vi "Main.vi"(11 "Module Admin":refnum<class "Delacor_lib_QMH_Module Admin.lvclass">) -> ()   [LabVIEW 2021, in "Host Main.lvlib"]
doc: "This template is based off of the Queued Message Handler design pattern and the Queued Message Handler project template that ships with LabVIEW.\n\nThe main difference is that the queue is private to this module and communication between modules is performed via Broadcast and Request events.\n\nRequest events are wrapped in public API methods and are handled in the Event Handling Loop (EHL) of this VI. Any module can register for Broadcast events sent by this module. The EHL generates messages based on user interface actions.\n\nThe Message Handling Loop (MHL) processes messages generated by the EHL, or by other messages. The messages are string values, so new messages can be added easily to the Message Cases case structure in the MHL. Each message cluster can also provide an optional value for Message Data, which is a variant that can be converted to whatever message-specific data is required.\n_____\nBased on DQMH Project Template 7.0.1.1316."
uses:
  Host Main.lvlib
  <vilib>/Delacor/Delacor QMH/Libraries/Module Admin_class/Delacor_lib_QMH_Module Admin.lvclass
  Analog Output/Controls/AO JSON Data Cluster.ctl
  Analog Output/Controls/AO Interface Data Cluster.ctl
  Analog Output/Controls/AO Channel Configuration Cluster.ctl
  Analog Output/Controls/AO Timing Cluster.ctl
  Digital Output/Controls/DIO Configuration cluster.ctl
  Digital Output/Controls/DIO Interface Data.ctl
  Digital Output/SubVIs/Digital Dynamic Cluster.ctl
  Module Data--cluster.ctl
  Host/Controls/Host - GUI Data Cluster.ctl
  Host/Async JSON Cluster.ctl
  Host/Async Interface Data Cluster.ctl
  Async Serial/Controls/Async Serial Configuration Cluster.ctl
  Async Serial/Controls/Async Frame Info Cluster.ctl
  Async Serial/Controls/Async Message Info Cluster.ctl
  Host/Controls/Host Data Cluster.ctl
  Main Engine/Controls/Main Engine CPU Info.ctl
  <vilib>/Wovalab/Utilities/Helper Loop Periodic Timing/Helper Loop Periodic Timing.lvclass/Helper Loop Periodic Timing.ctl
  Host-Control's/Module ID Action Enum.ctl
  Host-Control's/RT Exec FGV Action.ctl
  <vilib>/Delacor/Delacor QMH/Libraries/Message Queue_class/Delacor_lib_QMH_Message Queue.lvclass/Delacor_lib_QMH_Message Queue.ctl
  Stop Argument--cluster.ctl
  <vilib>/Delacor/Delacor QMH/Libraries/Module Admin_class/Delacor_lib_QMH_Module Admin.lvclass/Delacor_lib_QMH_Module Admin.ctl
  <vilib>/Utility/miscctls.llb/LVPointTypeDef.ctl
  Launch RT Acq Argument--cluster.ctl
  Host-Control's/DTT Test folder Name's.ctl
  Host-Control's/HW Name Enum.ctl
  <vilib>/Delacor/Delacor QMH/Libraries/Message Queue_class/Delacor_lib_QMH_Enqueue Message (Single).vi
  <vilib>/Delacor/Delacor QMH/Libraries/Module Admin_class/Delacor_lib_QMH_Get External Launch.vi
  <vilib>/Wovalab/Utilities/Helper Loop Periodic Timing/U32 Max Value--constant.vi
  <vilib>/Wovalab/Utilities/Helper Loop Periodic Timing/Update Last Execution Time.vi
  <vilib>/addons/_JKI.lib/Serialization/JSON/Library/Flatten To JSON String.vi
  <vilib>/Wovalab/Utilities/Helper Loop Periodic Timing/Helper Loop Periodic Timing.lvclass
  <vilib>/Delacor/Delacor QMH/Libraries/Message Queue_class/Delacor_lib_QMH_Message Queue.lvclass
  RT Acquisition Engine/RT Acquisition Engine.lvlib
  Test Configuration/Test Configuration.lvlib
  Test Panel/Test Panel.lvlib
  Configuration/Configuration.lvlib
  Hardware Selection/Hardware Selection.lvlib
  <userlib>/_OpenG.lib/appcontrol/appcontrol.llb/openg_application_control.lvlib
  RT Acquisition Engine/Clone Registration/Clone Registration.lvlib
  TCP-IP Engine/Clone Registration/Clone Registration.lvlib
  TCP-IP Engine/TCP-IP Engine.lvlib
  AS-Configuration/AS-Configuration.lvlib
  <vilib>/Utility/TDMS File Viewer/NI_TDMS File Viewer.lvlib
  Safety/Safety.lvlib
panel:
  in  "Hardware Selection":bool
  in  "AI 2":T1[](array[typedef]) {"Interface Data"."Timing"."sample mode" items=["Finite Samples"=10178, "Continuous Samples"=10123, "Hardware Timed Single Point"=12522]}
  out "Capsule-4":bool
  out "Capsule-2":bool
  out "Capsule-1":bool
  in  "DO":T5[](array[typedef])=[{"Interface"="DIO", "Interface Data"={"Command"="Configure", "SubCmd"="DO", "Frequency"=500, "Data"=[{"Channel"="Mod1/port0/line0", "Data"=[0], "Identification Name"=""}, {"Channel"="Mod1/port0/line1", "Data"=[0], "Identification Name"=""}, {"Channel"="Mod1/port0/line2", "Data"=[0], "Identification Name"=""}, {"Channel"="Mod1/port0/line3", "Data"=[0], "Identification Name"=""}, {"Channel"="Mod1/port0/line4", "Data"=[0], "Identification Name"=""}, {"Channel"="Mod1/port0/line5", "Data"=[0], "Identification Name"=""}, {"Channel"="Mod1/port0/line6", "Data"=[0], "Identification Name"=""}, {"Channel"="Mod1/port0/line7", "Data"=[0], "Identification Name"=""}, {"Channel"="Mod1/port0/line8", "Data"=[0], "Identification Name"=""}, {"Channel"="Mod1/port0/line9", "Data"=[0], "Identification Name"=""}, {"Channel"="Mod1/port0/line10", "Data"=[0], "Identification Name"=""}, {"Channel"="Mod1/port0/line11", "Data"=[0], "Identification Name"=""}, {"Channel"="Mod1/port0/line12", "Data"=[0], "Identification Name"=""}, {"Channel"="Mod1/port0/line13", "Data"=[0], "Identification Name"=""}, {"Channel"="Mod1/port0/line14", "Data"=[0], "Identification Name"=""}, {"Channel"="Mod1/port0/line15", "Data"=[0], "Identification Name"=""}, {"Channel"="Mod1/port0/line16", "Data"=[0], "Identification Name"=""}, {"Channel"="Mod1/port0/line17", "Data"=[0], "Identification Name"=""}, {"Channel"="Mod1/port0/line18", "Data"=[0], "Identification Name"=""}, {"Channel"="Mod1/port0/line19", "Data"=[0], "Identification Name"=""}, {"Channel"="Mod1/port0/line20", "Data"=[0], "Identification Name"=""}, {"Channel"="Mod1/port0/line21", "Data"=[0], "Identification Name"=""}, {"Channel"="Mod1/port0/line22", "Data"=[0], "Identification Name"=""}, {"Channel"="Mod1/port0/line23", "Data"=[0], "Identification Name"=""}, {"Channel"="Mod1/port0/line24", "Data"=[0], "Identification Name"=""}, {"Channel"="Mod1/port0/line25", "Data"=[0], "Identification Name"=""}, {"Channel"="Mod1/port0/line26", "Data"=[0], "Identification Name"=""}, {"Channel"="Mod1/port0/line27", "Data"=[0], "Identification Name"=""}, {"Channel"="Mod1/port0/line28", "Data"=[0], "Identification Name"=""}, {"Channel"="Mod1/port0/line29", "Data"=[0], "Identification Name"=""}, {"Channel"="Mod1/port0/line30", "Data"=[0], "Identification Name"=""}, {"Channel"="Mod1/port0/line31", "Data"=[0], "Identification Name"=""}]}}, {"Interface"="DIO", "Interface Data"={"Command"="Configure", "SubCmd"="DO", "Frequency"=500, "Data"=[{"Channel"="Mod1/port0/line0", "Data"=[0], "Identification Name"=""}, {"Channel"="Mod1/port0/line1", "Data"=[0], "Identification Name"=""}, {"Channel"="Mod1/port0/line2", "Data"=[0], "Identification Name"=""}, {"Channel"="Mod1/port0/line3", "Data"=[0], "Identification Name"=""}, {"Channel"="Mod1/port0/line4", "Data"=[0], "Identification Name"=""}, {"Channel"="Mod1/port0/line5", "Data"=[0], "Identification Name"=""}, {"Channel"="Mod1/port0/line6", "Data"=[0], "Identification Name"=""}, {"Channel"="Mod1/port0/line7", "Data"=[0], "Identification Name"=""}, {"Channel"="Mod1/port0/line8", "Data"=[0], "Identification Name"=""}, {"Channel"="Mod1/port0/line9", "Data"=[0], "Identification Name"=""}, {"Channel"="Mod1/port0/line10", "Data"=[0], "Identification Name"=""}, {"Channel"="Mod1/port0/line11", "Data"=[0], "Identification Name"=""}, {"Channel"="Mod1/port0/line12", "Data"=[0], "Identification Name"=""}, {"Channel"="Mod1/port0/line13", "Data"=[0], "Identification Name"=""}, {"Channel"="Mod1/port0/line14", "Data"=[0], "Identification Name"=""}, {"Channel"="Mod1/port0/line15", "Data"=[0], "Identification Name"=""}, {"Channel"="Mod1/port0/line16", "Data"=[0], "Identification Name"=""}, {"Channel"="Mod1/port0/line17", "Data"=[0], "Identification Name"=""}, {"Channel"="Mod1/port0/line18", "Data"=[0], "Identification Name"=""}, {"Channel"="Mod1/port0/line19", "Data"=[0], "Identification Name"=""}, {"Channel"="Mod1/port0/line20", "Data"=[0], "Identification Name"=""}, {"Channel"="Mod1/port0/line21", "Data"=[0], "Identification Name"=""}, {"Channel"="Mod1/port0/line22", "Data"=[0], "Identification Name"=""}, {"Channel"="Mod1/port0/line23", "Data"=[0], "Identification Name"=""}, {"Channel"="Mod1/port0/line24", "Data"=[0], "Identification Name"=""}, {"Channel"="Mod1/port0/line25", "Data"=[0], "Identification Name"=""}, {"Channel"="Mod1/port0/line26", "Data"=[0], "Identification Name"=""}, {"Channel"="Mod1/port0/line27", "Data"=[0], "Identification Name"=""}, {"Channel"="Mod1/port0/line28", "Data"=[0], "Identification Name"=""}, {"Channel"="Mod1/port0/line29", "Data"=[0], "Identification Name"=""}, {"Channel"="Mod1/port0/line30", "Data"=[0], "Identification Name"=""}, {"Channel"="Mod1/port0/line31", "Data"=[0], "Identification Name"=""}, {"Channel"="Mod2/port0/line0", "Data"=[0], "Identification Name"=""}, {"Channel"="Mod2/port0/line1", "Data"=[0], "Identification Name"=""}, {"Channel"="Mod2/port0/line2", "Data"=[0], "Identification Name"=""}, {"Channel"="Mod2/port0/line3", "Data"=[0], "Identification Name"=""}, {"Channel"="Mod2/port0/line4", "Data"=[0], "Identification Name"=""}, {"Channel"="Mod2/port0/line5", "Data"=[0], "Identification Name"=""}, {"Channel"="Mod2/port0/line6", "Data"=[0], "Identification Name"=""}, {"Channel"="Mod2/port0/line7", "Data"=[0], "Identification Name"=""}, {"Channel"="Mod2/port0/line8", "Data"=[0], "Identification Name"=""}]}}, {"Interface"="DIO", "Interface Data"={"Command"="Configure", "SubCmd"="DO", "Frequency"=500, "Data"=[{"Channel"="Mod1/port0/line0", "Data"=[0], "Identification Name"=""}, {"Channel"="Mod1/port0/line1", "Data"=[0], "Identification Name"=""}, {"Channel"="Mod1/port0/line2", "Data"=[0], "Identification Name"=""}, {"Channel"="Mod1/port0/line3", "Data"=[0], "Identification Name"=""}, {"Channel"="Mod1/port0/line4", "Data"=[0], "Identification Name"=""}, {"Channel"="Mod1/port0/line5", "Data"=[0], "Identification Name"=""}, {"Channel"="Mod1/port0/line6", "Data"=[], "Identification Name"=""}, {"Channel"="Mod1/port0/line7", "Data"=[0], "Identification Name"=""}, {"Channel"="Mod1/port0/line8", "Data"=[0], "Identification Name"=""}, {"Channel"="Mod1/port0/line9", "Data"=[0], "Identification Name"=""}, {"Channel"="Mod1/port0/line10", "Data"=[0], "Identification Name"=""}, {"Channel"="Mod1/port0/line11", "Data"=[0], "Identification Name"=""}, {"Channel"="Mod1/port0/line12", "Data"=[0], "Identification Name"=""}, {"Channel"="Mod1/port0/line13", "Data"=[0], "Identification Name"=""}, {"Channel"="Mod1/port0/line14", "Data"=[0], "Identification Name"=""}, {"Channel"="Mod1/port0/line15", "Data"=[0], "Identification Name"=""}, {"Channel"="Mod1/port0/line16", "Data"=[0], "Identification Name"=""}, {"Channel"="Mod1/port0/line17", "Data"=[0], "Identification Name"=""}, {"Channel"="Mod1/port0/line18", "Data"=[0], "Identification Name"=""}, {"Channel"="Mod1/port0/line19", "Data"=[0], "Identification Name"=""}, {"Channel"="Mod1/port0/line20", "Data"=[0], "Identification Name"=""}, {"Channel"="Mod1/port0/line21", "Data"=[0], "Identification Name"=""}, {"Channel"="Mod1/port0/line22", "Data"=[0], "Identification Name"=""}, {"Channel"="Mod1/port0/line23", "Data"=[0], "Identification Name"=""}, {"Channel"="Mod1/port0/line24", "Data"=[0], "Identification Name"=""}, {"Channel"="Mod1/port0/line25", "Data"=[0], "Identification Name"=""}, {"Channel"="Mod1/port0/line26", "Data"=[0], "Identification Name"=""}, {"Channel"="Mod1/port0/line27", "Data"=[0], "Identification Name"=""}, {"Channel"="Mod1/port0/line28", "Data"=[0], "Identification Name"=""}, {"Channel"="Mod1/port0/line29", "Data"=[0], "Identification Name"=""}, {"Channel"="Mod1/port0/line30", "Data"=[0], "Identification Name"=""}, {"Channel"="Mod1/port0/line31", "Data"=[0], "Identification Name"=""}]}}, {"Interface"="DIO", "Interface Data"={"Command"="Configure", "SubCmd"="DO", "Frequency"=500, "Data"=[{"Channel"="Mod1/port0/line0", "Data"=[0], "Identification Name"=""}, {"Channel"="Mod1/port0/line1", "Data"=[0], "Identification Name"=""}, {"Channel"="Mod1/port0/line2", "Data"=[0], "Identification Name"=""}, {"Channel"="Mod1/port0/line3", "Data"=[0], "Identification Name"=""}, {"Channel"="Mod1/port0/line4", "Data"=[0], "Identification Name"=""}, {"Channel"="Mod1/port0/line5", "Data"=[0], "Identification Name"=""}, {"Channel"="Mod1/port0/line6", "Data"=[0], "Identification Name"=""}, {"Channel"="Mod1/port0/line7", "Data"=[0], "Identification Name"=""}, {"Channel"="Mod1/port0/line8", "Data"=[0], "Identification Name"=""}, {"Channel"="Mod1/port0/line9", "Data"=[0], "Identification Name"=""}, {"Channel"="Mod1/port0/line10", "Data"=[0], "Identification Name"=""}, {"Channel"="Mod1/port0/line11", "Data"=[0], "Identification Name"=""}, {"Channel"="Mod1/port0/line12", "Data"=[0], "Identification Name"=""}, {"Channel"="Mod1/port0/line13", "Data"=[0], "Identification Name"=""}, {"Channel"="Mod1/port0/line14", "Data"=[0], "Identification Name"=""}, {"Channel"="Mod1/port0/line15", "Data"=[0], "Identification Name"=""}, {"Channel"="Mod1/port0/line16", "Data"=[0], "Identification Name"=""}, {"Channel"="Mod1/port0/line17", "Data"=[0], "Identification Name"=""}, {"Channel"="Mod1/port0/line18", "Data"=[0], "Identification Name"=""}, {"Channel"="Mod1/port0/line19", "Data"=[0], "Identification Name"=""}, {"Channel"="Mod1/port0/line20", "Data"=[0], "Identification Name"=""}, {"Channel"="Mod1/port0/line21", "Data"=[0], "Identification Name"=""}, {"Channel"="Mod1/port0/line22", "Data"=[0], "Identification Name"=""}, {"Channel"="Mod1/port0/line23", "Data"=[0], "Identification Name"=""}, {"Channel"="Mod1/port0/line24", "Data"=[0], "Identification Name"=""}, {"Channel"="Mod1/port0/line25", "Data"=[0], "Identification Name"=""}, {"Channel"="Mod1/port0/line26", "Data"=[0], "Identification Name"=""}, {"Channel"="Mod1/port0/line27", "Data"=[0], "Identification Name"=""}, {"Channel"="Mod1/port0/line28", "Data"=[0], "Identification Name"=""}, {"Channel"="Mod1/port0/line29", "Data"=[0], "Identification Name"=""}, {"Channel"="Mod1/port0/line30", "Data"=[0], "Identification Name"=""}, {"Channel"="Mod1/port0/line31", "Data"=[0], "Identification Name"=""}]}}, {"Interface"="DIO", "Interface Data"={"Command"="Configure", "SubCmd"="DO", "Frequency"=500, "Data"=[{"Channel"="Mod1/port0/line0", "Data"=[0], "Identification Name"=""}, {"Channel"="Mod1/port0/line1", "Data"=[0], "Identification Name"=""}, {"Channel"="Mod1/port0/line2", "Data"=[0], "Identification Name"=""}, {"Channel"="Mod1/port0/line3", "Data"=[0], "Identification Name"=""}, {"Channel"="Mod1/port0/line4", "Data"=[0], "Identification Name"=""}, {"Channel"="Mod1/port0/line5", "Data"=[0], "Identification Name"=""}, {"Channel"="Mod1/port0/line6", "Data"=[0], "Identification Name"=""}, {"Channel"="Mod1/port0/line7", "Data"=[0], "Identification Name"=""}, {"Channel"="Mod1/port0/line8", "Data"=[0], "Identification Name"=""}, {"Channel"="Mod1/port0/line9", "Data"=[0], "Identification Name"=""}, {"Channel"="Mod1/port0/line10", "Data"=[0], "Identification Name"=""}, {"Channel"="Mod1/port0/line11", "Data"=[0], "Identification Name"=""}, {"Channel"="Mod1/port0/line12", "Data"=[0], "Identification Name"=""}, {"Channel"="Mod1/port0/line13", "Data"=[0], "Identification Name"=""}, {"Channel"="Mod1/port0/line14", "Data"=[0], "Identification Name"=""}, {"Channel"="Mod1/port0/line15", "Data"=[0], "Identification Name"=""}, {"Channel"="Mod1/port0/line16", "Data"=[0], "Identification Name"=""}, {"Channel"="Mod1/port0/line17", "Data"=[0], "Identification Name"=""}, {"Channel"="Mod1/port0/line18", "Data"=[0], "Identification Name"=""}, {"Channel"="Mod1/port0/line19", "Data"=[0], "Identification Name"=""}, {"Channel"="Mod1/port0/line20", "Data"=[0], "Identification Name"=""}, {"Channel"="Mod1/port0/line21", "Data"=[0], "Identification Name"=""}, {"Channel"="Mod1/port0/line22", "Data"=[0], "Identification Name"=""}, {"Channel"="Mod1/port0/line23", "Data"=[0], "Identification Name"=""}, {"Channel"="Mod1/port0/line24", "Data"=[0], "Identification Name"=""}, {"Channel"="Mod1/port0/line25", "Data"=[0], "Identification Name"=""}, {"Channel"="Mod1/port0/line26", "Data"=[0], "Identification Name"=""}, {"Channel"="Mod1/port0/line27", "Data"=[0], "Identification Name"=""}, {"Channel"="Mod1/port0/line28", "Data"=[0], "Identification Name"=""}, {"Channel"="Mod1/port0/line29", "Data"=[0], "Identification Name"=""}, {"Channel"="Mod1/port0/line30", "Data"=[0], "Identification Name"=""}, {"Channel"="Mod1/port0/line31", "Data"=[0], "Identification Name"=""}]}}, {"Interface"="DIO", "Interface Data"={"Command"="Configure", "SubCmd"="DO", "Frequency"=500, "Data"=[{"Channel"="Mod1/port0/line0", "Data"=[0], "Identification Name"=""}, {"Channel"="Mod1/port0/line1", "Data"=[0], "Identification Name"=""}, {"Channel"="Mod1/port0/line2", "Data"=[0], "Identification Name"=""}, {"Channel"="Mod1/port0/line3", "Data"=[0], "Identification Name"=""}, {"Channel"="Mod1/port0/line4", "Data"=[0], "Identification Name"=""}, {"Channel"="Mod1/port0/line5", "Data"=[0], "Identification Name"=""}, {"Channel"="Mod1/port0/line6", "Data"=[0], "Identification Name"=""}, {"Channel"="Mod1/port0/line7", "Data"=[0], "Identification Name"=""}, {"Channel"="Mod1/port0/line8", "Data"=[0], "Identification Name"=""}, {"Channel"="Mod1/port0/line9", "Data"=[0], "Identification Name"=""}, {"Channel"="Mod1/port0/line10", "Data"=[0], "Identification Name"=""}, {"Channel"="Mod1/port0/line11", "Data"=[0], "Identification Name"=""}, {"Channel"="Mod1/port0/line12", "Data"=[0], "Identification Name"=""}, {"Channel"="Mod1/port0/line13", "Data"=[0], "Identification Name"=""}, {"Channel"="Mod1/port0/line14", "Data"=[0], "Identification Name"=""}, {"Channel"="Mod1/port0/line15", "Data"=[0], "Identification Name"=""}, {"Channel"="Mod1/port0/line16", "Data"=[0], "Identification Name"=""}, {"Channel"="Mod1/port0/line17", "Data"=[0], "Identification Name"=""}, {"Channel"="Mod1/port0/line18", "Data"=[0], "Identification Name"=""}, {"Channel"="Mod1/port0/line19", "Data"=[0], "Identification Name"=""}, {"Channel"="Mod1/port0/line20", "Data"=[0], "Identification Name"=""}, {"Channel"="Mod1/port0/line21", "Data"=[0], "Identification Name"=""}, {"Channel"="Mod1/port0/line22", "Data"=[0], "Identification Name"=""}, {"Channel"="Mod1/port0/line23", "Data"=[0], "Identification Name"=""}, {"Channel"="Mod1/port0/line24", "Data"=[0], "Identification Name"=""}, {"Channel"="Mod1/port0/line25", "Data"=[0], "Identification Name"=""}, {"Channel"="Mod1/port0/line26", "Data"=[0], "Identification Name"=""}, {"Channel"="Mod1/port0/line27", "Data"=[0], "Identification Name"=""}, {"Channel"="Mod1/port0/line28", "Data"=[0], "Identification Name"=""}, {"Channel"="Mod1/port0/line29", "Data"=[0], "Identification Name"=""}, {"Channel"="Mod1/port0/line30", "Data"=[0], "Identification Name"=""}, {"Channel"="Mod1/port0/line31", "Data"=[0], "Identification Name"=""}, {"Channel"="Mod2/port0/line0", "Data"=[0], "Identification Name"=""}, {"Channel"="Mod2/port0/line1", "Data"=[0], "Identification Name"=""}, {"Channel"="Mod2/port0/line2", "Data"=[0], "Identification Name"=""}, {"Channel"="Mod2/port0/line3", "Data"=[0], "Identification Name"=""}, {"Channel"="Mod2/port0/line4", "Data"=[0], "Identification Name"=""}, {"Channel"="Mod2/port0/line5", "Data"=[0], "Identification Name"=""}, {"Channel"="Mod2/port0/line6", "Data"=[0], "Identification Name"=""}, {"Channel"="Mod2/port0/line7", "Data"=[0], "Identification Name"=""}, {"Channel"="Mod2/port0/line8", "Data"=[0], "Identification Name"=""}, {"Channel"="Mod2/port0/line9", "Data"=[0], "Identification Name"=""}, {"Channel"="Mod2/port0/line10", "Data"=[0], "Identification Name"=""}, {"Channel"="Mod2/port0/line11", "Data"=[0], "Identification Name"=""}, {"Channel"="Mod2/port0/line12", "Data"=[0], "Identification Name"=""}, {"Channel"="Mod2/port0/line13", "Data"=[0], "Identification Name"=""}, {"Channel"="Mod2/port0/line14", "Data"=[0], "Identification Name"=""}, {"Channel"="Mod2/port0/line15", "Data"=[0], "Identification Name"=""}, {"Channel"="Mod2/port0/line16", "Data"=[0], "Identification Name"=""}, {"Channel"="Mod2/port0/line17", "Data"=[0], "Identification Name"=""}, {"Channel"="Mod2/port0/line18", "Data"=[0], "Identification Name"=""}, {"Channel"="Mod2/port0/line19", "Data"=[0], "Identification Name"=""}, {"Channel"="Mod2/port0/line20", "Data"=[0], "Identification Name"=""}, {"Channel"="Mod2/port0/line21", "Data"=[0], "Identification Name"=""}, {"Channel"="Mod2/port0/line22", "Data"=[0], "Identification Name"=""}, {"Channel"="Mod2/port0/line23", "Data"=[0], "Identification Name"=""}, {"Channel"="Mod2/port0/line24", "Data"=[0], "Identification Name"=""}, {"Channel"="Mod2/port0/line25", "Data"=[0], "Identification Name"=""}, {"Channel"="Mod2/port0/line26", "Data"=[0], "Identification Name"=""}, {"Channel"="Mod2/port0/line27", "Data"=[0], "Identification Name"=""}, {"Channel"="Mod2/port0/line28", "Data"=[0], "Identification Name"=""}, {"Channel"="Mod2/port0/line29", "Data"=[0], "Identification Name"=""}, {"Channel"="Mod2/port0/line30", "Data"=[0], "Identification Name"=""}, {"Channel"="Mod2/port0/line31", "Data"=[0], "Identification Name"=""}]}}]
  in  "DI":T5[](array[typedef])=[{"Interface"="DIO", "Interface Data"={"Command"="Configure", "SubCmd"="DI", "Frequency"=500, "Data"=[{"Channel"="Mod3/port0/line0", "Data"=[0], "Identification Name"=""}, {"Channel"="Mod3/port0/line1", "Data"=[0], "Identification Name"=""}, {"Channel"="Mod3/port0/line2", "Data"=[0], "Identification Name"=""}, {"Channel"="Mod3/port0/line3", "Data"=[0], "Identification Name"=""}, {"Channel"="Mod3/port0/line4", "Data"=[0], "Identification Name"=""}, {"Channel"="Mod3/port0/line5", "Data"=[0], "Identification Name"=""}, {"Channel"="Mod3/port0/line6", "Data"=[0], "Identification Name"=""}, {"Channel"="Mod3/port0/line7", "Data"=[0], "Identification Name"=""}, {"Channel"="Mod3/port0/line8", "Data"=[0], "Identification Name"=""}, {"Channel"="Mod3/port0/line9", "Data"=[0], "Identification Name"=""}, {"Channel"="Mod3/port0/line10", "Data"=[0], "Identification Name"=""}, {"Channel"="Mod3/port0/line11", "Data"=[0], "Identification Name"=""}, {"Channel"="Mod3/port0/line12", "Data"=[0], "Identification Name"=""}, {"Channel"="Mod3/port0/line13", "Data"=[0], "Identification Name"=""}, {"Channel"="Mod3/port0/line14", "Data"=[0], "Identification Name"=""}, {"Channel"="Mod3/port0/line15", "Data"=[0], "Identification Name"=""}, {"Channel"="Mod3/port0/line16", "Data"=[0], "Identification Name"=""}, {"Channel"="Mod3/port0/line17", "Data"=[0], "Identification Name"=""}, {"Channel"="Mod3/port0/line18", "Data"=[0], "Identification Name"=""}, {"Channel"="Mod3/port0/line19", "Data"=[0], "Identification Name"=""}, {"Channel"="Mod3/port0/line20", "Data"=[0], "Identification Name"=""}, {"Channel"="Mod3/port0/line21", "Data"=[0], "Identification Name"=""}, {"Channel"="Mod3/port0/line22", "Data"=[0], "Identification Name"=""}, {"Channel"="Mod3/port0/line23", "Data"=[0], "Identification Name"=""}, {"Channel"="Mod3/port0/line24", "Data"=[0], "Identification Name"=""}, {"Channel"="Mod3/port0/line25", "Data"=[0], "Identification Name"=""}, {"Channel"="Mod3/port0/line26", "Data"=[0], "Identification Name"=""}, {"Channel"="Mod3/port0/line27", "Data"=[0], "Identification Name"=""}, {"Channel"="Mod3/port0/line28", "Data"=[0], "Identification Name"=""}, {"Channel"="Mod3/port0/line29", "Data"=[0], "Identification Name"=""}, {"Channel"="Mod3/port0/line30", "Data"=[0], "Identification Name"=""}, {"Channel"="Mod3/port0/line31", "Data"=[0], "Identification Name"=""}, {"Channel"="Mod4/port0/line0", "Data"=[0], "Identification Name"=""}, {"Channel"="Mod4/port0/line1", "Data"=[0], "Identification Name"=""}, {"Channel"="Mod4/port0/line2", "Data"=[0], "Identification Name"=""}, {"Channel"="Mod4/port0/line3", "Data"=[0], "Identification Name"=""}, {"Channel"="Mod4/port0/line4", "Data"=[0], "Identification Name"=""}, {"Channel"="Mod4/port0/line5", "Data"=[0], "Identification Name"=""}, {"Channel"="Mod4/port0/line6", "Data"=[0], "Identification Name"=""}, {"Channel"="Mod4/port0/line7", "Data"=[0], "Identification Name"=""}, {"Channel"="Mod4/port0/line8", "Data"=[0], "Identification Name"=""}, {"Channel"="Mod4/port0/line9", "Data"=[0], "Identification Name"=""}, {"Channel"="Mod4/port0/line10", "Data"=[0], "Identification Name"=""}, {"Channel"="Mod4/port0/line11", "Data"=[0], "Identification Name"=""}, {"Channel"="Mod4/port0/line12", "Data"=[0], "Identification Name"=""}, {"Channel"="Mod4/port0/line13", "Data"=[0], "Identification Name"=""}, {"Channel"="Mod4/port0/line14", "Data"=[0], "Identification Name"=""}, {"Channel"="Mod4/port0/line15", "Data"=[0], "Identification Name"=""}, {"Channel"="Mod4/port0/line16", "Data"=[0], "Identification Name"=""}, {"Channel"="Mod4/port0/line17", "Data"=[0], "Identification Name"=""}, {"Channel"="Mod4/port0/line18", "Data"=[0], "Identification Name"=""}, {"Channel"="Mod4/port0/line19", "Data"=[0], "Identification Name"=""}, {"Channel"="Mod4/port0/line20", "Data"=[0], "Identification Name"=""}, {"Channel"="Mod4/port0/line21", "Data"=[0], "Identification Name"=""}, {"Channel"="Mod4/port0/line22", "Data"=[0], "Identification Name"=""}, {"Channel"="Mod4/port0/line23", "Data"=[0], "Identification Name"=""}, {"Channel"="Mod4/port0/line24", "Data"=[0], "Identification Name"=""}, {"Channel"="Mod4/port0/line25", "Data"=[0], "Identification Name"=""}, {"Channel"="Mod4/port0/line26", "Data"=[0], "Identification Name"=""}, {"Channel"="Mod4/port0/line27", "Data"=[0], "Identification Name"=""}, {"Channel"="Mod4/port0/line28", "Data"=[0], "Identification Name"=""}, {"Channel"="Mod4/port0/line29", "Data"=[0], "Identification Name"=""}, {"Channel"="Mod4/port0/line30", "Data"=[0], "Identification Name"=""}, {"Channel"="Mod4/port0/line31", "Data"=[0], "Identification Name"=""}]}}, {"Interface"="DIO", "Interface Data"={"Command"="", "SubCmd"="DI", "Frequency"=500, "Data"=[]}}, {"Interface"="DIO", "Interface Data"={"Command"="Configure", "SubCmd"="DI", "Frequency"=500, "Data"=[{"Channel"="Mod3/port0/line0", "Data"=[0], "Identification Name"=""}, {"Channel"="Mod3/port0/line1", "Data"=[0], "Identification Name"=""}, {"Channel"="Mod3/port0/line2", "Data"=[0], "Identification Name"=""}, {"Channel"="Mod3/port0/line3", "Data"=[0], "Identification Name"=""}, {"Channel"="Mod3/port0/line4", "Data"=[0], "Identification Name"=""}, {"Channel"="Mod3/port0/line5", "Data"=[0], "Identification Name"=""}, {"Channel"="Mod3/port0/line6", "Data"=[0], "Identification Name"=""}, {"Channel"="Mod3/port0/line7", "Data"=[0], "Identification Name"=""}, {"Channel"="Mod3/port0/line8", "Data"=[0], "Identification Name"=""}, {"Channel"="Mod3/port0/line9", "Data"=[0], "Identification Name"=""}, {"Channel"="Mod3/port0/line10", "Data"=[0], "Identification Name"=""}, {"Channel"="Mod3/port0/line11", "Data"=[0], "Identification Name"=""}, {"Channel"="Mod3/port0/line12", "Data"=[0], "Identification Name"=""}, {"Channel"="Mod3/port0/line13", "Data"=[0], "Identification Name"=""}, {"Channel"="Mod3/port0/line14", "Data"=[0], "Identification Name"=""}, {"Channel"="Mod3/port0/line15", "Data"=[0], "Identification Name"=""}, {"Channel"="Mod3/port0/line16", "Data"=[0], "Identification Name"=""}, {"Channel"="Mod3/port0/line17", "Data"=[0], "Identification Name"=""}, {"Channel"="Mod3/port0/line18", "Data"=[0], "Identification Name"=""}, {"Channel"="Mod3/port0/line19", "Data"=[0], "Identification Name"=""}, {"Channel"="Mod3/port0/line20", "Data"=[0], "Identification Name"=""}, {"Channel"="Mod3/port0/line21", "Data"=[0], "Identification Name"=""}, {"Channel"="Mod3/port0/line22", "Data"=[0], "Identification Name"=""}, {"Channel"="Mod3/port0/line23", "Data"=[0], "Identification Name"=""}, {"Channel"="Mod3/port0/line24", "Data"=[0], "Identification Name"=""}, {"Channel"="Mod3/port0/line25", "Data"=[0], "Identification Name"=""}, {"Channel"="Mod3/port0/line26", "Data"=[0], "Identification Name"=""}, {"Channel"="Mod3/port0/line27", "Data"=[0], "Identification Name"=""}, {"Channel"="Mod3/port0/line28", "Data"=[0], "Identification Name"=""}, {"Channel"="Mod3/port0/line29", "Data"=[0], "Identification Name"=""}, {"Channel"="Mod3/port0/line30", "Data"=[0], "Identification Name"=""}, {"Channel"="Mod3/port0/line31", "Data"=[0], "Identification Name"=""}, {"Channel"="Mod4/port0/line0", "Data"=[0], "Identification Name"=""}, {"Channel"="Mod4/port0/line1", "Data"=[0], "Identification Name"=""}, {"Channel"="Mod4/port0/line2", "Data"=[0], "Identification Name"=""}, {"Channel"="Mod4/port0/line3", "Data"=[0], "Identification Name"=""}, {"Channel"="Mod4/port0/line4", "Data"=[0], "Identification Name"=""}, {"Channel"="Mod4/port0/line5", "Data"=[0], "Identification Name"=""}, {"Channel"="Mod4/port0/line6", "Data"=[0], "Identification Name"=""}, {"Channel"="Mod4/port0/line7", "Data"=[0], "Identification Name"=""}, {"Channel"="Mod4/port0/line8", "Data"=[0], "Identification Name"=""}, {"Channel"="Mod4/port0/line9", "Data"=[0], "Identification Name"=""}, {"Channel"="Mod4/port0/line10", "Data"=[0], "Identification Name"=""}, {"Channel"="Mod4/port0/line11", "Data"=[0], "Identification Name"=""}, {"Channel"="Mod4/port0/line12", "Data"=[0], "Identification Name"=""}, {"Channel"="Mod4/port0/line13", "Data"=[0], "Identification Name"=""}, {"Channel"="Mod4/port0/line14", "Data"=[0], "Identification Name"=""}, {"Channel"="Mod4/port0/line15", "Data"=[0], "Identification Name"=""}, {"Channel"="Mod4/port0/line16", "Data"=[0], "Identification Name"=""}, {"Channel"="Mod4/port0/line17", "Data"=[0], "Identification Name"=""}, {"Channel"="Mod4/port0/line18", "Data"=[0], "Identification Name"=""}, {"Channel"="Mod4/port0/line19", "Data"=[0], "Identification Name"=""}, {"Channel"="Mod4/port0/line20", "Data"=[0], "Identification Name"=""}, {"Channel"="Mod4/port0/line21", "Data"=[0], "Identification Name"=""}, {"Channel"="Mod4/port0/line22", "Data"=[0], "Identification Name"=""}, {"Channel"="Mod4/port0/line23", "Data"=[0], "Identification Name"=""}, {"Channel"="Mod4/port0/line24", "Data"=[0], "Identification Name"=""}, {"Channel"="Mod4/port0/line25", "Data"=[0], "Identification Name"=""}, {"Channel"="Mod4/port0/line26", "Data"=[0], "Identification Name"=""}, {"Channel"="Mod4/port0/line27", "Data"=[0], "Identification Name"=""}, {"Channel"="Mod4/port0/line28", "Data"=[0], "Identification Name"=""}, {"Channel"="Mod4/port0/line29", "Data"=[0], "Identification Name"=""}, {"Channel"="Mod4/port0/line30", "Data"=[0], "Identification Name"=""}, {"Channel"="Mod4/port0/line31", "Data"=[0], "Identification Name"=""}]}}, {"Interface"="DIO", "Interface Data"={"Command"="Configure", "SubCmd"="DI", "Frequency"=500, "Data"=[]}}, {"Interface"="DIO", "Interface Data"={"Command"="Configure", "SubCmd"="DI", "Frequency"=500, "Data"=[]}}, {"Interface"="DIO", "Interface Data"={"Command"="Configure", "SubCmd"="DI", "Frequency"=500, "Data"=[]}}]
  in  "AI":T1[](array[typedef]) {"Interface Data"."Timing"."sample mode" items=["Finite Samples"=10178, "Continuous Samples"=10123, "Hardware Timed Single Point"=12522]}
  in  "RT-IP":string[](array[string])
  in  "Customize \nControl Names":bool
  out "Safety":bool
  out "Release":bool
  in  "Log in":bool
  in  "Test  configuration":bool
  in  "Release Module Config":bool
  in  "Acquisition Module Configuration":bool
  in  "Offline Analysis":bool=TRUE
  in  "Automatic Sequence \nConfiguration":bool=TRUE
  out "sbRIO":bool
  out "Capsule-3":bool
  in  "Run Test":bool
  in  "User Manual":bool
  in  "About Us":bool
  out "error out":errorcluster
  out "Status":string
  in  "Simulate MHL Error":bool
  in  "Simulate EHL Error":bool
  # "IIT-M Drop Tower Test System"
  # "MAIN PANEL"
  # "Developed by SyncSols"
  # "All Rights Reserved | Copyright © 2024"
  # "CONNECTION STATUS"
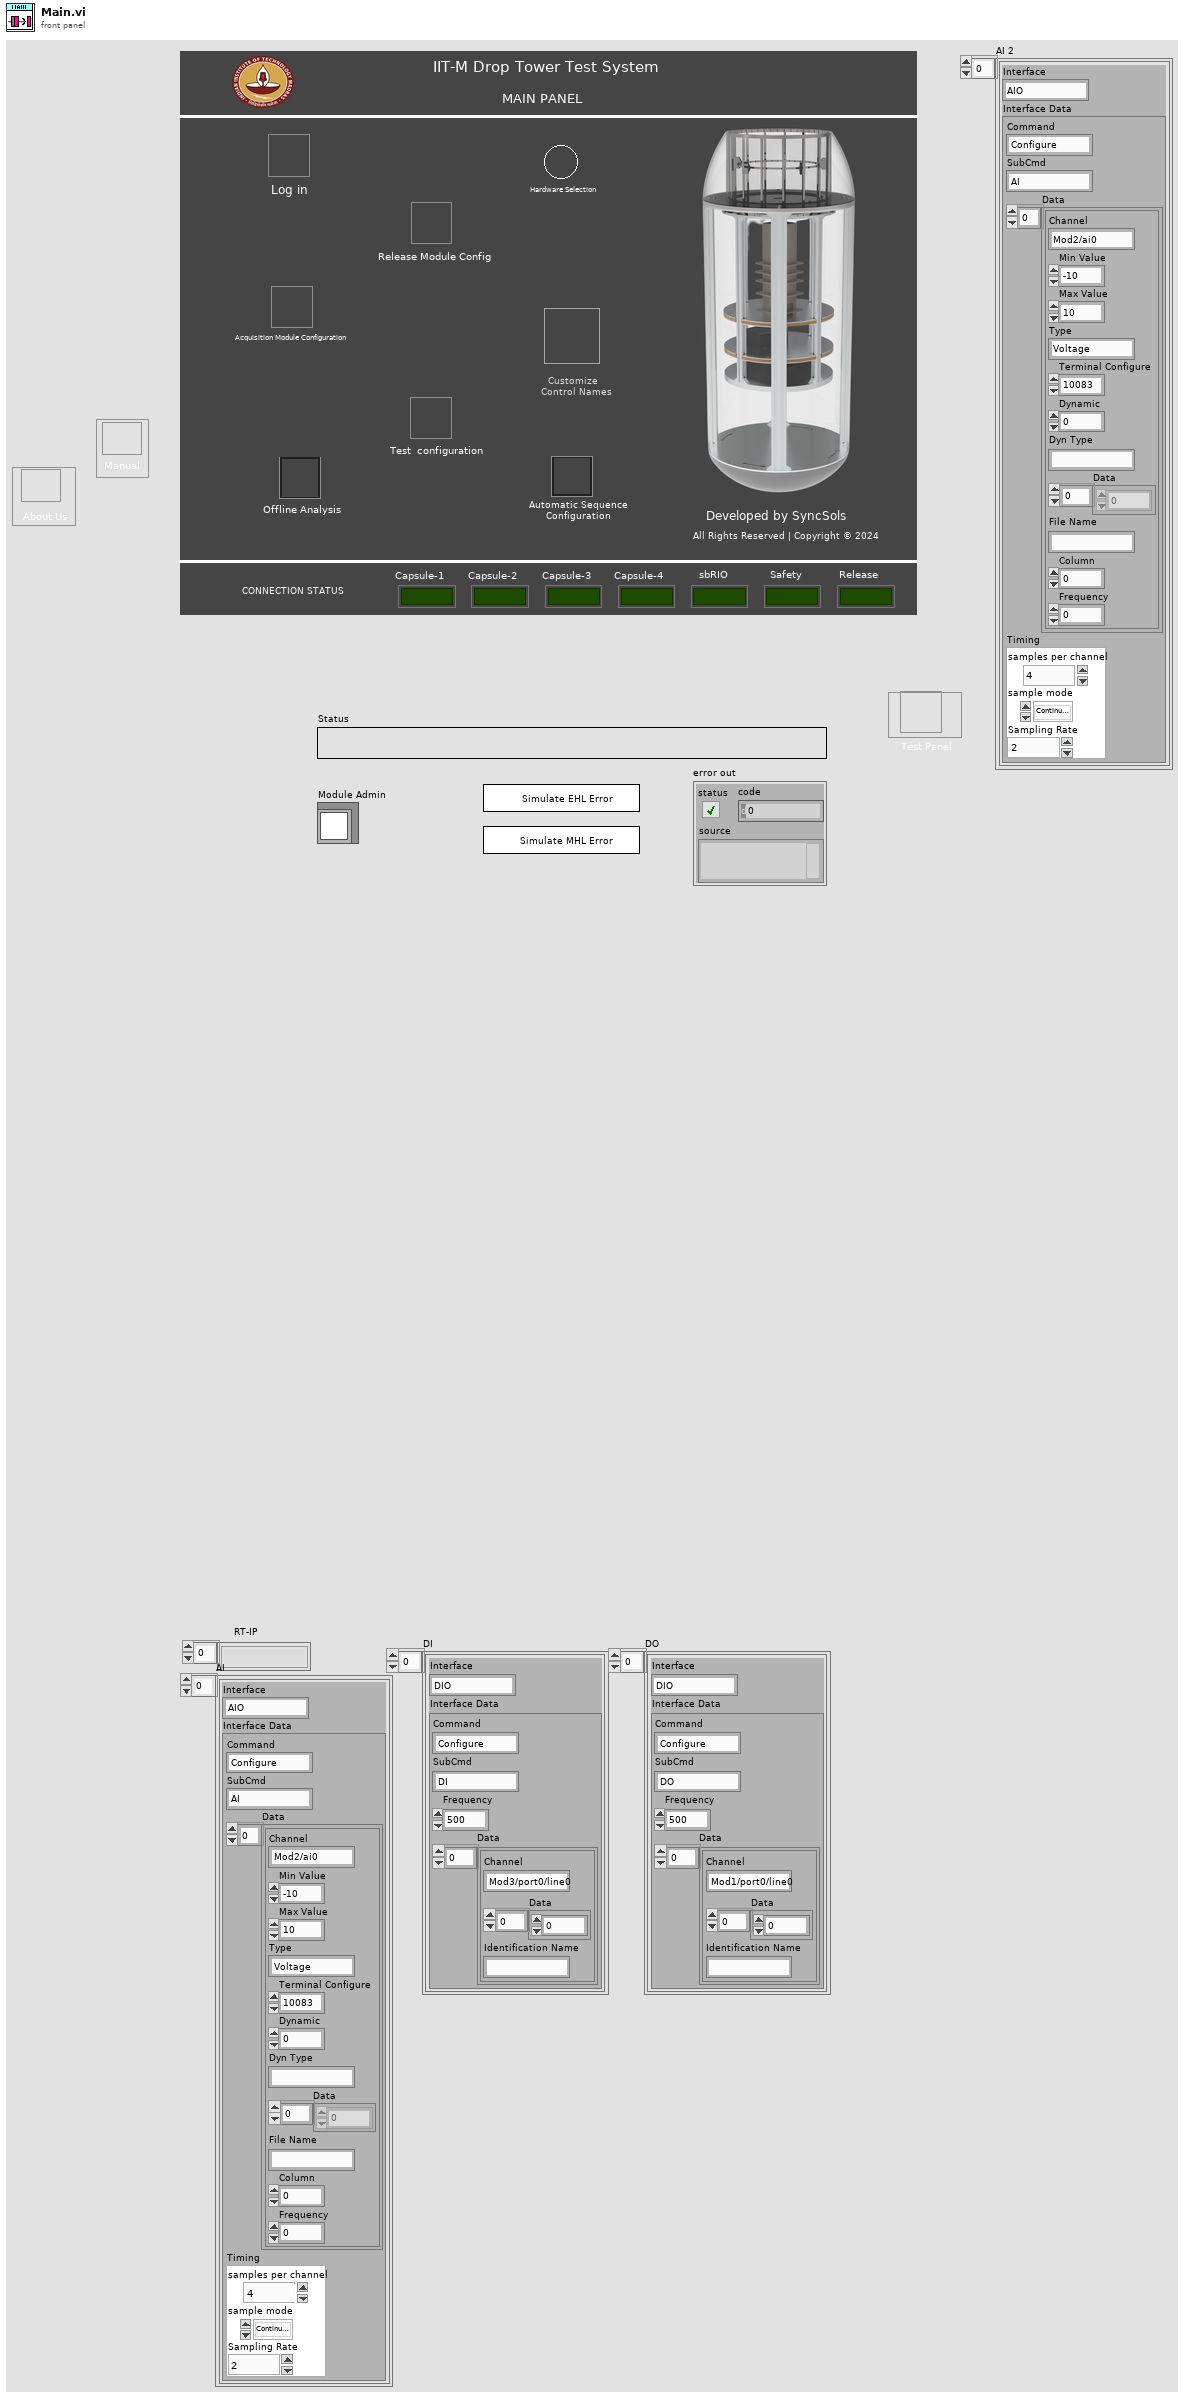
[diagram p1: front panel]
types:
  T1 = typedef "AO JSON Data Cluster.ctl" = cluster{"Interface":string, "Interface Data":T2}
  T2 = typedef "AO Interface Data Cluster.ctl" = cluster{"Command":string, "SubCmd":string, "Data":T3[], "Timing":T4}
  T3 = typedef "AO Channel Configuration Cluster.ctl" = cluster{"Channel":string, "Min Value":dbl, "Max Value":dbl, "Type":string, "Terminal Configure":u16, "Dynamic":u8, "Dyn Type":string, "Data":dbl[], "File Name":string, "Column":i32, "Frequency":dbl}
  T4 = typedef "AO Timing Cluster.ctl" = cluster{"samples per channel":i32, "sample mode":i32, "Sampling Rate":dbl}
  T5 = typedef "DIO Configuration cluster.ctl" = cluster{"Interface":string, "Interface Data":T6}
  T6 = typedef "DIO Interface Data.ctl" = cluster{"Command":string, "SubCmd":string, "Frequency":u16, "Data":T7[]}
  T7 = typedef "Digital Dynamic Cluster.ctl" = cluster{"Channel":string, "Data":u8[], "Identification Name":string}
  T8 = typedef "Test Configuration.lvlib/Broadcast Events--cluster.ctl" = cluster{"Module Did Init":refnum<user-event>, "Status Updated":refnum<user-event>, "Error Reported":refnum<user-event>, "Module Did Stop":refnum<user-event>, "Update Module Execution Status":refnum<user-event>}
  T9 = typedef "Hardware Selection.lvlib/Broadcast Events--cluster.ctl" = cluster{"Module Did Init":refnum<user-event>, "Status Updated":refnum<user-event>, "Error Reported":refnum<user-event>, "Module Did Stop":refnum<user-event>, "Update Module Execution Status":refnum<user-event>, "Selected RT HW":refnum<user-event>}
  T10 = typedef "AS-Configuration.lvlib/Broadcast Events--cluster.ctl" = cluster{"Module Did Init":refnum<user-event>, "Status Updated":refnum<user-event>, "Error Reported":refnum<user-event>, "Module Did Stop":refnum<user-event>, "Update Module Execution Status":refnum<user-event>}
  T11 = typedef "Configuration.lvlib/Broadcast Events--cluster.ctl" = cluster{"Module Did Init":refnum<user-event>, "Status Updated":refnum<user-event>, "Error Reported":refnum<user-event>, "Module Did Stop":refnum<user-event>, "Update Module Execution Status":refnum<user-event>}
  T12 = typedef "Host Main.lvlib/Request Events--cluster.ctl" = cluster{"Show Panel":refnum<user-event>, "Hide Panel":refnum<user-event>, "Get Module Execution Status":refnum<user-event>, "Show Diagram":refnum<user-event>, "Private":cluster{"Launch RT Acq":refnum<user-event>}, "Stop Module":refnum<user-event>, "Launch TP":refnum<user-event>}
  T13 = typedef "Host Main.lvlib/Module Data--cluster.ctl" = cluster{"Status":string, "Data Cluster":T14, "RT-Acq Id":i32[], "RT-IP":string[]}
  T14 = typedef "Host - GUI Data Cluster.ctl" = cluster{"VI References":refnum<vi>[], "Addresses":string[], "Pilot":bool, "DO Data":cluster{"Names":string[], "Data":bool[]}[], "Access Restricted?":bool, "Pilot Control References":refnum<vi>[], "CoPilot Control References":refnum<vi>[], "cRIO Config":cluster{"AI":T1, "DI":T5, "DO":T5, "Async":T15}[], "datalog Q":refnum<queue>, "PS_P":T20, "PS_S":T20, "IDE_P":T20, "IDE_S":T20, "PDE_P":T20, "PDE_S":T20, "GUI References":cluster{"Control Names":string[], "Control References":refnum<vi>[]}, "GUI Data":string[][], "TCP - Serial":string[][], "TCP-Serial Q":refnum<queue>, "TCP Serial Ref":refnum<vi>[], "Data Sets":dbl[][], "Last Data":dbl[], "Alarm Data":cluster{"Alarm Value":dbl, "Data Index":i32, "DO target Index":i32, "DO Index":i32, "DI target Index":i32, "DI Index":i32}[], "DI Data":cluster{bool[]}[], "Ack Data":cluster{"Alarm Value":dbl, "Data Index":i32, "DO target Index":i32, "DO Index":i32, "DI target Index":i32, "DI Index":i32}[], "Buzzer Data":cluster{"Alarm Value":dbl, "Data Index":i32, "DO target Index":i32, "DO Index":i32, "DI target Index":i32, "DI Index":i32}[], "Pilot DO":cluster{"Data":i32[]}[], "Co-Pilot DO":cluster{"Data":i32[]}[], "System Down?":bool, "Log Data":dbl[], "Update Array":i32[][], "MCC Data Log":dbl[], "MCC Data Not":refnum<notifier>, "Thruster control":refnum<vi>[], "waga notifier out":refnum<notifier>, "Wago  log":sgl[], "Thruster Cont":dbl[], "Cam Cont":bool[], "PDE_P TH Cont":cluster{"COM 10":dbl, "COM 11":dbl, "COM 12":dbl, "COM 13":dbl}, "PDE_S TH Cont":cluster{"COM 10":dbl, "COM 11":dbl, "COM 12":dbl, "COM 13":dbl}}
  T15 = typedef "Async JSON Cluster.ctl" = cluster{"Interface":string, "Interface Data":T16}
  T16 = typedef "Async Interface Data Cluster.ctl" = cluster{"Command":string, "SubCmd":string, "Data":T17[]}
  T17 = typedef "Async Serial Configuration Cluster.ctl" = cluster{"Port":string, "Minor Frame Freq":u16, "Minor Frame Count":u16, "Frame Info":T18[], "Sensor Type":u16, "OIM Address":u16}
  T18 = typedef "Async Frame Info Cluster.ctl" = cluster{"Frame ID":u16, "Message Info":T19[]}
  T19 = typedef "Async Message Info Cluster.ctl" = cluster{"Message":u8[], "Message Name":string}
  T20 = typedef "Host Data Cluster.ctl" = cluster{"AI":dbl[], "DI":bool[], "DO":bool[], "Serial":string[][], "CPU":T21, "Stop":bool, "DO Channel":string[]}
  T21 = typedef "Main Engine CPU Info.ctl" = cluster{"Total Load":u32[], "Interrupt Load":u32[], "Total Physical":dbl, "Free Physical":dbl, "Primary Disk Capacity":dbl, "Primary Disk Free":dbl}
  T22 = typedef "Module ID Action Enum.ctl" = enum16{"Init", "Insert", "Get a ID", "Get all ID"}
  T23 = typedef "RT Exec FGV Action.ctl" = enum16{"Init", "Insert", "Get a Exec?", "Get All Exec?"}
  T24 = enum32{"invalid lock state", "Not Locked", "Locked (No Password)", "Password-protected"}
  T25 = typedef "Host Main.lvlib/Stop Argument--cluster.ctl" = cluster{"Origin":string, "Exit via Stop Module Req?":bool, "Wait for Module to stop?":bool}
  T26 = typedef "LVPointTypeDef.ctl" = cluster{"Horizontal":i16, "Vertical":i16}
  T27 = enum32{"Invalid", "Standard", "Closed", "Hidden", "Minimized", "Maximized"}
  T28 = typedef "DTT Test folder Name's.ctl" = enum16{"Event Log", "Auto Sequence Configuration", "Channel Configuration's", "Test Data's"}
  T29 = typedef "HW Name Enum.ctl" = enum16{"Capsule-1", "Capsule-2", "Capsule-3", "Capsule-4", "sb-RIO", "Safety", "Release"}
  T30 = typedef "RT Acquisition Engine.lvlib/Broadcast Events--cluster.ctl" = cluster{"Module Did Init":refnum<user-event>, "Status Updated":refnum<user-event>, "Error Reported":refnum<user-event>, "Module Did Stop":refnum<user-event>, "Update Module Execution Status":refnum<user-event>, "RT Connection Status":refnum<user-event>, "Tx RT Hardware Info":refnum<user-event>, "DO Data's":refnum<user-event>, "AI-Info":refnum<user-event>, "Logging Completed":refnum<user-event>}
  T31 = typedef "Test Panel.lvlib/Broadcast Events--cluster.ctl" = cluster{"Module Did Init":refnum<user-event>, "Status Updated":refnum<user-event>, "Error Reported":refnum<user-event>, "Module Did Stop":refnum<user-event>, "Update Module Execution Status":refnum<user-event>}
  T32 = typedef "Safety.lvlib/Broadcast Events--cluster.ctl" = cluster{"Module Did Init":refnum<user-event>, "Status Updated":refnum<user-event>, "Error Reported":refnum<user-event>, "Did Something":refnum<user-event>, "Module Did Stop":refnum<user-event>, "Update Module Execution Status":refnum<user-event>, "Connection Status":refnum<user-event>}
  T33 = typedef "Host Main.lvlib/Launch RT Acq Argument--cluster.ctl" = cluster{"HW-IP":string[], "HW-Name":string[], "AI":T1[], "DI":T5[], "DO":T5[]}
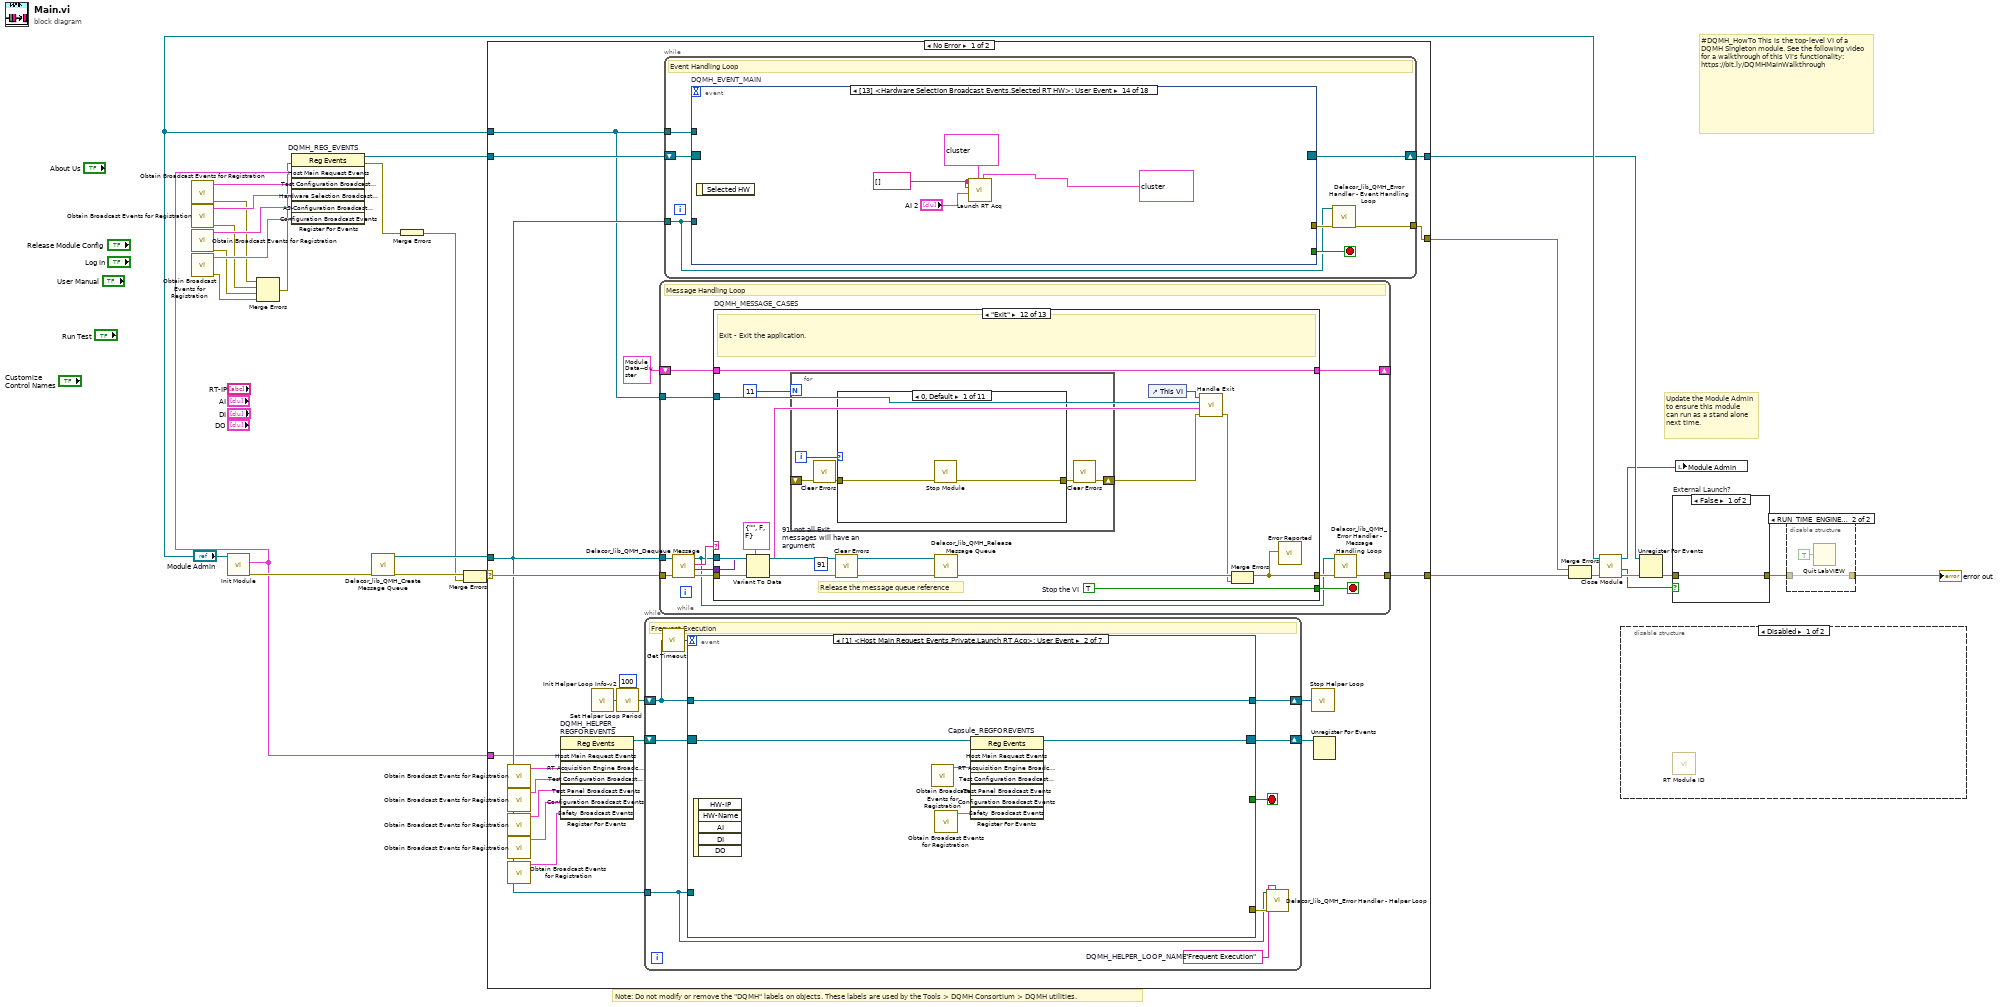
[diagram p0: block diagram]
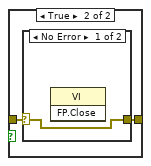
[diagram p4: hidden frame]
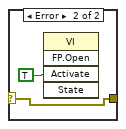
[diagram p5: hidden frame]
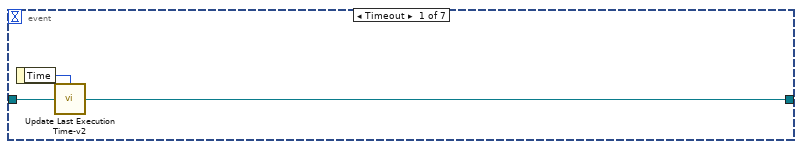
[diagram p6: hidden frame]
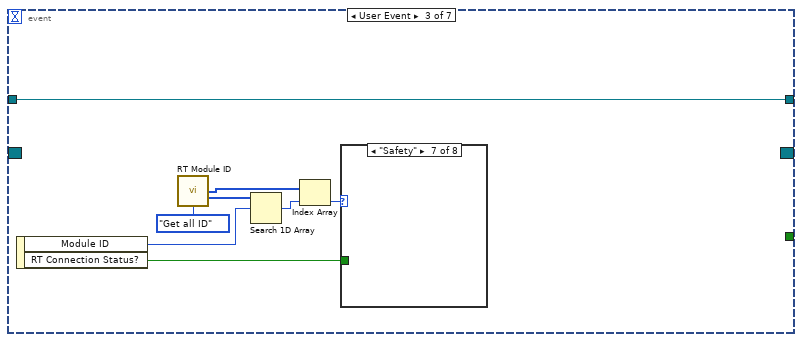
[diagram p7: hidden frame]
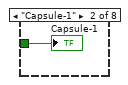
[diagram p9: hidden frame]
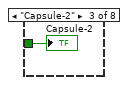
[diagram p10: hidden frame]
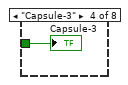
[diagram p11: hidden frame]
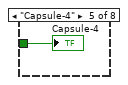
[diagram p12: hidden frame]
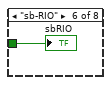
[diagram p13: hidden frame]
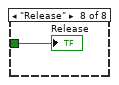
[diagram p14: hidden frame]
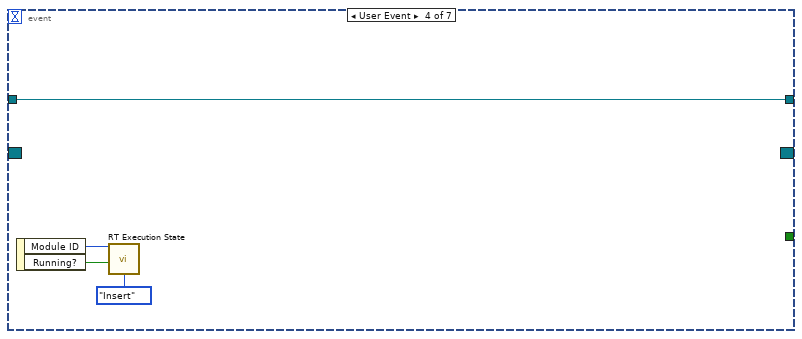
[diagram p15: hidden frame]
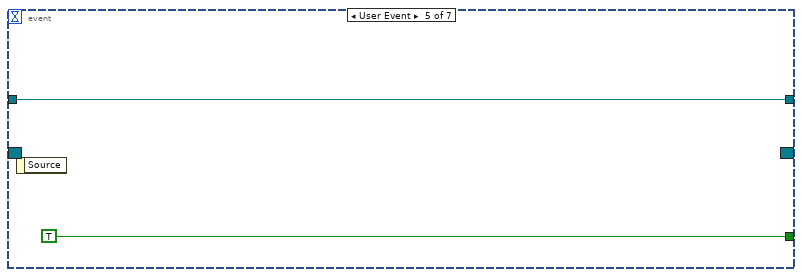
[diagram p16: hidden frame]
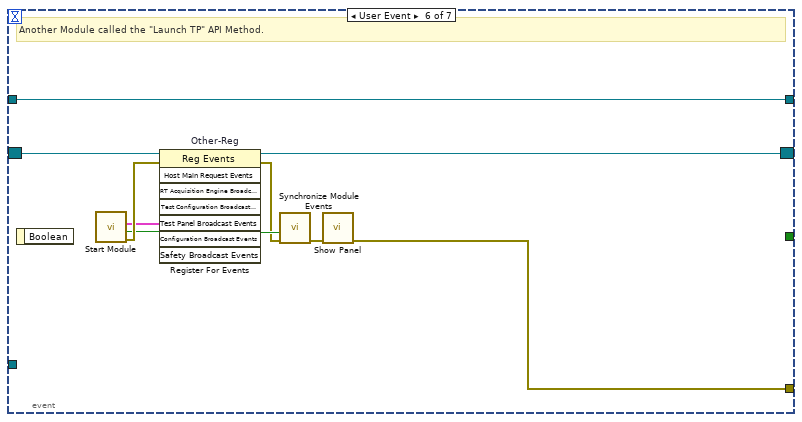
[diagram p17: hidden frame]
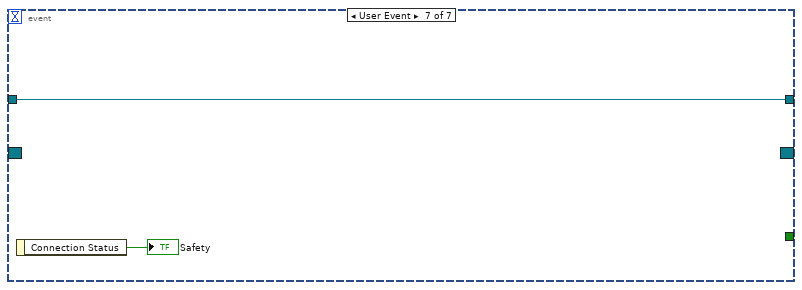
[diagram p18: hidden frame]
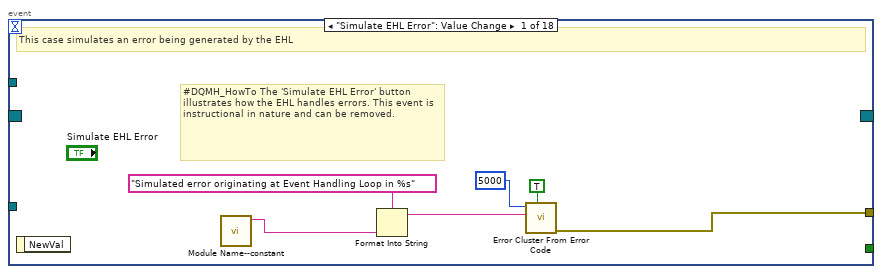
[diagram p19: hidden frame]
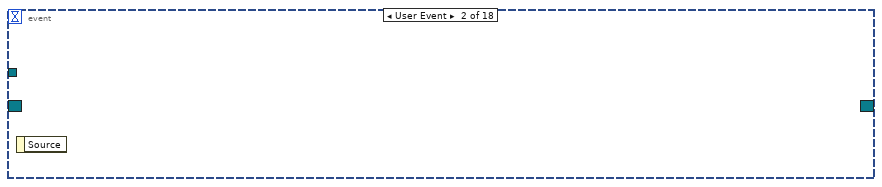
[diagram p20: hidden frame]
diagram:
  # "#DQMH_HowTo This is the top-level VI of a DQMH Singleton module. See the following video for a walkthrough of this VI's functionality: https://bit.ly/DQMHMainWalkthrough"
  # "Note: Do not modify or remove the \"DQMH\" labels on objects. These labels are used by the Tools > DQMH Consortium > DQMH utilities."
  # "Update the Module Admin to ensure this module can run as a stand alone next time."
  n1 = call "Obtain Broadcast Events for Registration.vi"() -> ("error out"=w5:errorcluster, "Test Configuration Broadcast Events"=w13:T8)  [unwired: 9 in, 1 out]
  n2 = call "Obtain Broadcast Events for Registration.vi"() -> ("error out"=w4:errorcluster, "Hardware Selection Broadcast Events"=w9:T9)  [unwired: 9 in, 1 out]
  n3 = call "Obtain Broadcast Events for Registration.vi"() -> ("error out"=w2:errorcluster, "AS-Configuration Broadcast Events"=w7:T10)  [unwired: 9 in, 1 out]
  n4 = call "Obtain Broadcast Events for Registration.vi"() -> ("error out"=w1:errorcluster, "Configuration Broadcast Events"=w6:T11)  [unwired: 9 in, 1 out]
  n5 = call "Init Module.vi"("Singleton Module Admin in"="Module Admin") -> ("error out"=w28:errorcluster, "Host Main Request Events"=w14:T12, "Singleton Module Admin out"=w21:refnum<class "Delacor_lib_QMH_Module Admin.lvclass">)  [unwired: 8 in]
  n6 = Merge Errors(w5, w4, w2, w1) -> (w3:errorcluster)
  n7 = register-events "DQMH_REG_EVENTS"(error in=w3, w14, w13, w9, w7, w6) -> (reference out=w19:refnum<event-registration>, error out=w8:errorcluster)  [unwired: 1 in]
  n8 = call <vilib>:"Delacor_lib_QMH_Create Message Queue.vi"("error in"=w28) -> ("error out"=w23:errorcluster, "Message Queue"=w18:refnum<class "Delacor_lib_QMH_Message Queue.lvclass">)  [unwired: 9 in]
  n9 = Merge Errors(w8) -> (w12:errorcluster)
  n10 = Merge Errors(w23, w12) -> (w22:errorcluster)
  n11 = case shown="No Error" w22 {
    selector: w22 -> [w47 w412]
    tunnel: [w49 w411] -> w29
    tunnel: [w46 w410] -> w20
    tunnel: w19 -> [w44 w410]
    tunnel: w18 -> [w43 w405]
    tunnel: [w48 _] -> w26
    tunnel: w21 -> [w42 w406]
    tunnel: w14 -> [w41 _]
    frame No Error {
      n12 = call "Obtain Broadcast Events for Registration.vi"() -> ("RT Acquisition Engine Broadcast Events"=w34:T30)  [unwired: 9 in, 2 out]
      n13 = call "Obtain Broadcast Events for Registration.vi"() -> ("Test Configuration Broadcast Events"=w33:T8)  [unwired: 9 in, 2 out]
      n14 = call "Obtain Broadcast Events for Registration.vi"() -> ("Test Panel Broadcast Events"=w32:T31)  [unwired: 9 in, 2 out]
      n15 = call "Obtain Broadcast Events for Registration.vi"() -> ("Configuration Broadcast Events"=w31:T11)  [unwired: 9 in, 2 out]
      n16 = call "Obtain Broadcast Events for Registration.vi"() -> ("Safety Broadcast Events"=w30:T32)  [unwired: 9 in, 2 out]
      n17 = register-events "DQMH_HELPER_REGFOREVENTS"(w41, w34, w33, w32, w31, w30) -> (reference out=w39:refnum<event-registration>)  [unwired: 2 in, 1 out]
      n18 = call <vilib>:"Init Helper Loop Info-v2.vi"() -> ("Helper Loop Periodic Timing"=w37:refnum<class "Helper Loop Periodic Timing.lvclass">)  [unwired: 1 in]
      n19 = call <vilib>:"Set Helper Loop Period.vi"("Period (ms)"=100, "Helper Loop Periodic Timing in"=w37) -> ("Helper Loop Periodic Timing out"=w38:refnum<class "Helper Loop Periodic Timing.lvclass">)  [unwired: 13 in]
      n20 = while "DQMH_HELPER_LOOP" {
        shift-right: [w58] -> w36
        shift-left: w38 -> [w51]
        shift-right: [w56] -> w40
        shift-left: w39 -> [w57]
        tunnel: w43 -> [w54]
        stop <- w50 stop-if-true
        w53 = "Frequent Execution"  # DQMH_HELPER_LOOP_NAME
        # "Frequent Execution"
        n21 = call <vilib>:"Get Timeout.vi"("Helper Loop Periodic Timing"=w51) -> ("Timeout (ms)"=w52:i32)  [unwired: 12 in, 2 out]
        n22 = event "DQMH_HELPER_EVENT_STRUCTURE" shown="[1] <Host Main Request Events.Private.Launch RT Acq>: User Event" {
          selector: w57 -> [_ w65 _ _ _ w94 _]
          dyn-events: [_ w64 _ _ _ w87 _] -> w56
          timeout: w52 -> [_ _ _ _ _ _ _]
          tunnel: w51 -> [w60 w66 w74 w84 w86 w95 w97]
          tunnel: [w59 w66 w74 w84 w86 w95 w97] -> w58
          tunnel: [_ _ _ _ TRUE _ _] -> w50
          tunnel: [_ _ _ _ _ w88 _] -> w55
          tunnel: w54 -> [_ _ _ _ _ _ _]
          event Timeout {
            n23 = event-data() -> ("Time"=w61:u32)  [unwired: 1 in]
            n24 = call <vilib>:"Update Last Execution Time-v2.vi"("Time"=w61, "Helper Loop Periodic Timing in"=w60) -> ("Helper Loop Periodic Timing out"=w59:refnum<class "Helper Loop Periodic Timing.lvclass">)  [unwired: 12 in, 1 out]
          }
          event User Event {
            n25 = event-data() -> ()  [unwired: 1 in, 5 out]
            n26 = call "Obtain Broadcast Events for Registration.vi"() -> ("RT Acquisition Engine Broadcast Events"=w63:T30)  [unwired: 9 in, 2 out]
            n27 = call "Obtain Broadcast Events for Registration.vi"() -> ("Safety Broadcast Events"=w62:T32)  [unwired: 9 in, 2 out]
            n28 = register-events "Capsule_REGFOREVENTS"(reference=w65, w63, w62) -> (reference out=w64:refnum<event-registration>)  [unwired: 5 in, 1 out]
          }
          event User Event {
            n29 = event-data() -> ("Module ID"=w71:i32, "RT Connection Status?"=w73:bool)  [unwired: 1 in]
            n30 = call "RT Module ID.vi"("Action"=Module_ID_Action_Enum."Get all ID") -> ("All HW Name Out"=w68:T29[], "All HW-ID Out"=w69:i32[])  [unwired: 11 in, 2 out]
            n31 = Search 1D Array(1D array=w69, element=w71) -> (index of element=w70:i32)  [unwired: 1 in]
            n32 = Index Array(array=w68, index=w70) -> (element=w67:T29)
            n33 = case shown="\"Safety\"" w67 {
              tunnel: w73 -> [_ w75 w76 w77 w78 w79 _ w80]
              frame Default {
              }
              frame "Capsule-1" {
                "Capsule-1" <- w75
              }
              frame "Capsule-2" {
                "Capsule-2" <- w76
              }
              frame "Capsule-3" {
                "Capsule-3" <- w77
              }
              frame "Capsule-4" {
                "Capsule-4" <- w78
              }
              frame "sb-RIO" {
                "sbRIO" <- w79
              }
              frame "Safety" {
              }
              frame "Release" {
                "Release" <- w80
              }
            }
          }
          event User Event {
            n34 = event-data() -> ("Module ID"=w82:i32, "Running?"=w81:bool)  [unwired: 1 in]
            n35 = call "RT Execution State.vi"("Module ID In"=w82, "Exec State?"=w81, "Action"=RT_Exec_FGV_Action."Insert") -> ()  [unwired: 9 in, 4 out]
          }
          event User Event {
            n36 = event-data() -> ()  [unwired: 1 in, 1 out]
          }
          event User Event {
            # "Another Module called the \"Launch TP\" API Method."
            n37 = event-data() -> ()  [unwired: 1 in, 1 out]
            n38 = call "Start Module.vi"() -> ("error out"=w93:errorcluster, "Wait for Event Sync?"=w92:bool, "Test Panel Broadcast Events"=w91:T31)  [unwired: 8 in, 1 out]
            n39 = register-events "Other-Reg"(reference=w94, error in=w93, w91) -> (reference out=w87:refnum<event-registration>, error out=w90:errorcluster)  [unwired: 5 in]
            n40 = call "Synchronize Module Events.vi"("error in"=w90, "Wait for Event Sync?"=w92) -> ("error out"=w89:errorcluster)  [unwired: 9 in]
            n41 = call "Show Panel.vi"("error in"=w89) -> ("error out"=w88:errorcluster)  [unwired: 10 in]
          }
          event User Event {
            n42 = event-data() -> ("Connection Status"=→"Safety":bool)  [unwired: 1 in]
          }
        }
        n43 = call-dynamic "Delacor_lib_QMH_Error Handler - Helper Loop.vi"("Error Debug"=w53, "error in"=w55, "Message Queue in"=w54) -> ()  [unwired: 7 in, 2 out]
      }
      n44 = while {
        tunnel: w43 -> [w214]
        shift-right: [w222] -> _
        shift-left: T13 {"Status"="", "Data Cluster"={"VI References"=[], "Addresses"=[], "Pilot"=FALSE, "DO Data"=[], "Access Restricted?"=FALSE, "Pilot Control References"=[], "CoPilot Control References"=[], "cRIO Config"=[], "datalog Q"=refnum, "PS_P"={"AI"=[], "DI"=[], "DO"=[], "Serial"=[], "CPU"={"Total Load"=[], "Interrupt Load"=[], "Total Physical"=0.0, "Free Physical"=0.0, "Primary Disk Capacity"=0.0, "Primary Disk Free"=0.0}, "Stop"=FALSE, "DO Channel"=[]}, "PS_S"={"AI"=[], "DI"=[], "DO"=[], "Serial"=[], "CPU"={"Total Load"=[], "Interrupt Load"=[], "Total Physical"=0.0, "Free Physical"=0.0, "Primary Disk Capacity"=0.0, "Primary Disk Free"=0.0}, "Stop"=FALSE, "DO Channel"=[]}, "IDE_P"={"AI"=[], "DI"=[], "DO"=[], "Serial"=[], "CPU"={"Total Load"=[], "Interrupt Load"=[], "Total Physical"=0.0, "Free Physical"=0.0, "Primary Disk Capacity"=0.0, "Primary Disk Free"=0.0}, "Stop"=FALSE, "DO Channel"=[]}, "IDE_S"={"AI"=[], "DI"=[], "DO"=[], "Serial"=[], "CPU"={"Total Load"=[], "Interrupt Load"=[], "Total Physical"=0.0, "Free Physical"=0.0, "Primary Disk Capacity"=0.0, "Primary Disk Free"=0.0}, "Stop"=FALSE, "DO Channel"=[]}, "PDE_P"={"AI"=[], "DI"=[], "DO"=[], "Serial"=[], "CPU"={"Total Load"=[], "Interrupt Load"=[], "Total Physical"=0.0, "Free Physical"=0.0, "Primary Disk Capacity"=0.0, "Primary Disk Free"=0.0}, "Stop"=FALSE, "DO Channel"=[]}, "PDE_S"={"AI"=[], "DI"=[], "DO"=[], "Serial"=[], "CPU"={"Total Load"=[], "Interrupt Load"=[], "Total Physical"=0.0, "Free Physical"=0.0, "Primary Disk Capacity"=0.0, "Primary Disk Free"=0.0}, "Stop"=FALSE, "DO Channel"=[]}, "GUI References"={"Control Names"=[], "Control References"=[]}, "GUI Data"=[], "TCP - Serial"=[], "TCP-Serial Q"=refnum, "TCP Serial Ref"=[], "Data Sets"=[], "Last Data"=[], "Alarm Data"=[], "DI Data"=[], "Ack Data"=[], "Buzzer Data"=[], "Pilot DO"=[], "Co-Pilot DO"=[], "System Down?"=FALSE, "Log Data"=[], "Update Array"=[], "MCC Data Log"=[], "MCC Data Not"=refnum, "Thruster control"=[refnum, refnum, refnum, refnum, refnum, refnum, refnum, refnum, refnum], "waga notifier out"=refnum, "Wago  log"=[], "Thruster Cont"=[0.0, 0.0, 0.0, 0.0, 0.0, 0.0, 0.0, 0.0, 0.0, 0.0, 0.0], "Cam Cont"=[FALSE, FALSE, FALSE, FALSE, FALSE, TRUE], "PDE_P TH Cont"={"COM 10"=0.0, "COM 11"=0.0, "COM 12"=0.0, "COM 13"=0.0}, "PDE_S TH Cont"={"COM 10"=0.0, "COM 11"=0.0, "COM 12"=0.0, "COM 13"=0.0}}, "RT-Acq Id"=[], "RT-IP"=[]} ("Data Cluster") -> [w223]
        tunnel: w47 -> [w225]
        tunnel: [w217] -> w49
        tunnel: w42 -> [w218]
        stop <- w221 stop-if-true
        # "Message Handling Loop"
        n45 = call-dynamic "Delacor_lib_QMH_Dequeue Message.vi"("error in"=w225, "Message Queue in"=w214) -> ("error out"=w224:errorcluster, "Message Data"=w219:variant, "Message"=w220:string, "Message Queue out"=w215:refnum<class "Delacor_lib_QMH_Message Queue.lvclass">)  [unwired: 6 in]
        n46 = case "DQMH_MESSAGE_CASES" shown="\"Exit\"" w220 {
          selector: w220 -> [_ _ _ _ _ _ _ _ _ _ _ _ w400]
          tunnel: w215 -> [w234 w264 _ _ _ _ _ _ _ _ w319 w344 _]
          tunnel: w224 -> [w251 w263 w268 w270 w279 w282 w293 w304 w306 w315 w326 w349 w403]
          tunnel: [w231 w262 w268 w270 w278 w281 w292 w303 w306 w314 w322 w345 w404] -> w216
          tunnel: w223 -> [w241 w266 w267 w269 w274 w280 w291 w302 w305 w312 w321 w336 w401]
          tunnel: [w240 w266 w267 w269 w273 w280 w291 w302 w305 w312 w321 w336 w401] -> w222
          tunnel: [_ _ _ _ _ _ _ _ _ _ _ w343 _] -> w221
          tunnel: w219 -> [_ _ _ _ w277 _ _ _ _ _ w320 w342 _]
          tunnel: w218 -> [w242 _ _ _ _ _ _ _ _ _ w318 w337 _]
          frame "Initialize" {
            w236 = "Initial Message" ("Initial Message")
            # "#CodeNeeded - Initialize the appearance of the front panel."
            # "#CodeNeeded - Initialize your state data here."
            # "Initialize - Any operation that needs to be done before the module can receive messages. Synchronize Caller Events.vi will inform Start Module.vi that the module has launched and is ready to receive messages. Module Did Init.vi will broadcast that the module initialized."
            n47 = call "Synchronize Caller Events.vi"("error in"=w251, "Singleton Module Admin in"=w242) -> ("error out"=w250:errorcluster, "Singleton Module Admin out"=w237:refnum<class "Delacor_lib_QMH_Module Admin.lvclass">)  [unwired: 8 in]
            n48 = property on="Property Node" class="Module Admin"(reference=w237) -> ("Accessors:External Launch"=w246:bool)  [unwired: 1 in, 2 out]
            n49 = Select(t=T27."Hidden" ("State"), s=w246, f=T27."Standard" ("State")) -> (s? t:f=w243:T27)
            n50 = control-ref of="This VI"() -> (w229:refnum<vi>)
            n51 = call "Module Name--constant.vi"() -> ("Module Name"=w249:string)  [unwired: 11 in]
            n52 = property on="Property Node" class="VI"(reference=w229, "Front Panel.Title"=w249) -> (reference out=w248:refnum<vi>, error out=w253:errorcluster)  [unwired: 1 in]
            n53 = call "Module Name--constant.vi"() -> ("Module Name"=w238:string)  [unwired: 11 in]
            n54 = invoke on="Invoke Node" class="VI" method="FP.Open"(reference=w248, error in=w253, "State"=w243) -> (reference out=w247:refnum<vi>, error out=w252:errorcluster)  [unwired: 2 in, 3 out]
            n55 = Bundle By Name(cluster=w241, "Status"=w236) -> (w240:T13)
            n56 = call "Module Did Init.vi"("error in"=w250, "Initialized?"=TRUE, "Origin"=w238) -> ("error out"=w233:errorcluster)  [unwired: 8 in]
            n57 = invoke on="Invoke Node" class="VI" method="FP.Center"(reference=w247, error in=w252) -> (reference out=w226:refnum<vi>, error out=w228:errorcluster)  [unwired: 1 in, 1 out]
            n58 = property on="Pane" class="Pane"("Origin"=T26 {"Horizontal"=0, "Vertical"=0}) -> ()  [unwired: 2 in, 2 out]
            n59 = call <vilib>:"Clear Errors.vi"("error in (no error)"=w228) -> ("error out"=w227:errorcluster)  [unwired: 5 in, 1 out]
            n60 = call <userlib>:"Fit VI window to Largest Dec__ogtk.vi"("error in (no error)"=w227, "VI Ref (calling VI)"=w226) -> ("error out"=w230:errorcluster)  [unwired: 4 in, 1 out]
            n61 = call <vilib>:"Clear Errors.vi"("error in (no error)"=w230) -> ()  [unwired: 5 in, 2 out]
            n62 = call-poly <vilib>:"Delacor_lib_QMH_Enqueue Message (poly).vi"("error in"=w233, "Message"="Init-1", "Message Queue in"=w234) -> ("error out"=w231:errorcluster)  [unwired: 7 in, 1 out]
            "Status" <- w236
          }
          frame "Init-1" {
            # "Separator -- The following cases handle messages specific to this Module."
            n63 = call "Folder Creation.vi"("Create New? (F)"=TRUE) -> ("error out"=w260:errorcluster)  [unwired: 12 in, 2 out]
            n64 = call "File Path's.vi"("Create New? (F)"=TRUE, "error in"=w260) -> ("error out"=w259:errorcluster)  [unwired: 12 in, 1 out]
            n65 = control-ref of="This VI"() -> (w261:refnum<vi>)
            n66 = call "RT Execution State.vi"("error in"=w259, "Action"=RT_Exec_FGV_Action."Init") -> ("error out"=w258:errorcluster)  [unwired: 10 in, 3 out]
            n67 = invoke on="Invoke Node" class="VI" method="Default Vals.Reinit All"(reference=w261) -> ()  [unwired: 2 in, 3 out]
            n68 = call "RT Module ID.vi"("error in"=w258, "Action"=Module_ID_Action_Enum."Init") -> ()  [unwired: 10 in, 4 out]
            n69 = call-poly <vilib>:"Delacor_lib_QMH_Enqueue Message (poly).vi"("error in"=w263, "Message"="Init-2", "Message Queue in"=w264) -> ("error out"=w262:errorcluster)  [unwired: 7 in, 1 out]
          }
          frame "Init-2" {
            # "Separator -- The following cases handle messages specific to this Module."
          }
          frame "---Module Specific---" {
            # "Separator -- The following cases handle messages specific to this Module."
          }
          frame "Launch RT Acq" {
            (unwired) T33 data[24185B] ("Launch RT Acq Argument")
            # "This request event will launch the RT Acquisition module's based on the Given Input's."
            n70 = Variant To Data(error in=w279, type=cluster{"RT-IP":string[], "RT-Module Id":i32[]} {"RT-IP"=[], "RT-Module Id"=[]}, Variant=w277) -> (data=w276:cluster{"RT-IP":string[], "RT-Module Id":i32[]}, error out=w278:errorcluster)
            n71 = Unbundle By Name(w276) -> ("RT-IP"=w272:string[], "RT-Module Id"=w271:i32[])
            n72 = Bundle By Name(cluster=w274, "RT-IP"=w272, "RT-Acq Id"=w271) -> (w273:T13)
            n73 = call "RT-Module Id's.vi"("RT-Module Id"=w271, "RT-IP"=w272) -> ()  [unwired: 9 in, 1 out]
          }
          frame "---Copy This Frame---" {
            # "Duplicate this frame when creating new messages.  Change this comment in the duplicated frame to describe this message."
            n74 = Merge Errors(w282) -> (w281:errorcluster)
          }
          frame "Launch Offline Analysis" {
            # "Duplicate this frame when creating new messages.  Change this comment in the duplicated frame to describe this message."
            n75 = call "Hide Panel.vi"() -> ("error out"=w284:errorcluster)  [unwired: 11 in]
            n76 = call "Folder Creation.vi"("error in"=w284, "Folder Name"=DTT_Test_folder_Name's."Test Data's") -> ("Selected Folder Path Out"=w290:path, "error out"=w285:errorcluster)  [unwired: 11 in, 1 out]
            n77 = call "File Dialog"("start path"=w290, "error in"=w285) -> ("selected path"=w286:path, "cancelled"=w288:bool, "error out"=w287:errorcluster)  [unwired: 10 in, 1 out]
            n78 = case shown="False" w288 {
              tunnel: w286 -> [w296 _]
              tunnel: w287 -> [w295 _]
              tunnel: [w294 _] -> w289
              frame False {
                n79 = call <vilib>:"TDMS - File Viewer (NXG Style).vi"("error in"=w295, "file in"=w296) -> ("error out"=w294:errorcluster)  [unwired: 8 in, 1 out]
              }
              frame True {
              }
            }
            n80 = call "Show Panel.vi"("error in"=w289) -> ()  [unwired: 10 in, 1 out]
            n81 = Merge Errors(w293) -> (w292:errorcluster)
          }
          frame "Stop RT Application's" {
            # "Duplicate this frame when creating new messages.  Change this comment in the duplicated frame to describe this message."
            n82 = call "RT Module ID.vi"("HW Name"=HW_Name_Enum."Capsule-4", "Action"=Module_ID_Action_Enum."Get a ID") -> ("Module Id Out"=w298:i32)  [unwired: 10 in, 3 out]
            n83 = call "Data to JSON string Conversion.vi"("Interface"="Exit") -> ("Cmd String"=w297:string)  [unwired: 9 in, 1 out]
            n84 = call "Write Data To the RT.vi"("Data In"=w297, "Module ID"=w298) -> ()  [unwired: 9 in, 1 out]
            n85 = Merge Errors(w304) -> (w303:errorcluster)
          }
          frame "---Exit and Error Handling---" {
            # "Separator - The following cases handle errors and exit messages."
          }
          frame "Simulate MHL Error" {
            # "#DQMH_HowTo The 'Simulate MHL Error' button  illustrates how the MHL handles errors. This event is instructional in nature and can be removed."
            # "Simulate an error occurring at the MHL"
            n86 = call "Module Name--constant.vi"() -> ("Module Name"=w308:string)  [unwired: 11 in]
            n87 = Format Into String(format string="Simulated error originating at Message Handling Loop in %s", w308) -> (resulting string=w309:string)  [unwired: 2 in, 1 out]
            n88 = call <vilib>:"Error Cluster From Error Code.vi"("show call chain? (False)"=TRUE, "error message (\"\")"=w309, "error code (0)"=5001) -> ("error out"=w313:errorcluster)  [unwired: 6 in]
            n89 = Merge Errors(w315, w313) -> (w314:errorcluster)
          }
          frame "Error" {
            # "#CodeRecommended - If the module is running in standalone mode (External Launch = FALSE), this code will pop up an error dialog and call the 'Exit' message if an error occurs. Add more fine-grained error management here."
            # "Error - Check the error message data and respond accordingly. This message is sent by the \"Error Handler\" VIs at the end of each loop in this application."
            n90 = Variant To Data(error in=w326, type=errorcluster {"status"=FALSE, "code"=0, "source"=""} ("error constant"), Variant=w320) -> (data=w316:errorcluster, error out=w324:errorcluster)
            n91 = property on="Property Node" class="Module Admin"(reference=w318) -> ("Accessors:External Launch"=w317:bool)  [unwired: 1 in, 2 out]
            n92 = local write "error out"(w316) -> ()
            n93 = call "Error Reported.vi"("Error"=w316) -> ()  [unwired: 10 in, 1 out]
            n94 = case shown="False" w317 {
              tunnel: [w331 _] -> w323
              tunnel: w319 -> [w329 _]
              tunnel: w316 -> [w330 _]
              frame False {
                n95 = disable-structure shown="Default" {
                  disable-tunnel: w330 -> [w332 _]
                  frame condition #0 (active) {
                    # "If the module is running standalone, then pop up an error dialog and call the \"Exit\" message."
                    n96 = call <vilib>:"Simple Error Handler.vi"("error in (no error)"=w332) -> ()  [unwired: 4 in, 5 out]
                  }
                  frame condition #1 {
                    # "To prevent the Simple Error Handler VI from being loaded (e.g. when deploying to a Real-Time target), add the Conditional Disable Symbol \"DQMH_Disable_SEH\" to your project and set it to TRUE."
                  }
                }
                n97 = call-poly <vilib>:"Delacor_lib_QMH_Enqueue Message (poly).vi"("Priority Message? (F)"=TRUE, "Message"="Exit", "Message Queue in"=w329) -> ("error out"=w331:errorcluster)  [unwired: 7 in, 1 out]
              }
              frame True {
                # "If the module was launched externally, calling the Error Reported broadcast VI is the only action performed by the \"Error\" message. The module's caller can then process the error appropriately."
              }
            }
            n98 = Merge Errors(w324, w323) -> (w322:errorcluster)
          }
          frame "Exit" {
            w341 = 91  # 91: not all Exit messages will have an argument
            w343 = TRUE  # Stop the VI
            # "Release the message queue reference"
            # "Exit - Exit the application."
            n99 = Variant To Data(error in=w349, type=T25 {"Origin"="", "Exit via Stop Module Req?"=FALSE, "Wait for Module to stop?"=FALSE} ("Stop Argument"), Variant=w342) -> (data=w339:T25, error out=w346:errorcluster)
            n100 = for {
              N: 11 -> [_]
              shift-right: [w351] -> w333
              shift-left: _ -> [w354]
              i -> [w353]
              n101 = call <vilib>:"Clear Errors.vi"("error in (no error)"=w354) -> ("error out"=w350:errorcluster)  [unwired: 5 in, 1 out]
              n102 = case shown="0, Default" w353 {
                tunnel: w350 -> [w356 w358 w359 w361 w363 w367 w375 w380 w385 w392 w394]
                tunnel: [w355 w357 w359 w360 w362 w365 w373 w380 w382 w392 w393] -> w352
                frame 0, Default {
                  n103 = call "Stop Module.vi"("error in"=w356) -> ("error out"=w355:errorcluster)  [unwired: 10 in]
                }
                frame 1 {
                  n104 = call "Stop Module.vi"("error in"=w358) -> ("error out"=w357:errorcluster)  [unwired: 10 in]
                }
                frame 2 {
                }
                frame 3 {
                  n105 = call "Stop Module.vi"("error in"=w361) -> ("error out"=w360:errorcluster)  [unwired: 10 in]
                }
                frame 4 {
                  n106 = call "Stop Module.vi"("error in"=w363) -> ("error out"=w362:errorcluster)  [unwired: 10 in]
                }
                frame 5 {
                  n107 = call "List Instances.vi"("error in"=w367) -> ("error out"=w366:errorcluster, "Module IDs"=w364:i32[])  [unwired: 6 in, 3 out]
                  n108 = for {
                    tunnel: w364 -> [w370] mode=indexing
                    shift-right: [w368] -> w365
                    shift-left: w366 -> [w369]
                    n109 = call "Stop Module.vi"("error in"=w369, "Wait for Module to stop? (F)"=TRUE, "Module ID"=w370) -> ("error out"=w368:errorcluster)  [unwired: 8 in]
                  }
                }
                frame 6 {
                  n110 = call "List Instances.vi"("error in"=w375) -> ("error out"=w374:errorcluster, "Module IDs"=w372:i32[])  [unwired: 6 in, 3 out]
                  n111 = for {
                    tunnel: w372 -> [w377] mode=indexing
                    shift-right: [w378] -> w373
                    shift-left: w374 -> [w379]
                    n112 = call "Stop Module.vi"("error in"=w379, "Wait for Module to stop? (F)"=TRUE, "Module ID"=w377) -> ("error out"=w378:errorcluster)  [unwired: 8 in]
                  }
                }
                frame 7 {
                }
                frame 8 {
                  n113 = call "RT Module ID.vi"("error in"=w385, "Action"=Module_ID_Action_Enum."Get all ID") -> ("All HW-ID Out"=w381:i32[], "error out"=w383:errorcluster)  [unwired: 10 in, 2 out]
                  n114 = for {
                    shift-right: [w387] -> w382
                    shift-left: w383 -> [w391]
                    tunnel: w381 -> [w389] mode=indexing
                    n115 = call <vilib>:"Clear Errors.vi"("error in (no error)"=w391) -> ("error out"=w386:errorcluster)  [unwired: 5 in, 1 out]
                    n116 = call "Stop Module.vi"("error in"=w386, "Wait for Module to stop? (F)"=TRUE, "Module ID"=w389) -> ("error out"=w390:errorcluster)  [unwired: 8 in]
                    n117 = call <vilib>:"Clear Errors.vi"("error in (no error)"=w390) -> ("error out"=w387:errorcluster)  [unwired: 5 in, 1 out]
                  }
                }
                frame 9 {
                }
                frame 10 {
                  n118 = call "Stop Module.vi"("error in"=w394) -> ("error out"=w393:errorcluster)  [unwired: 10 in]
                }
              }
              n119 = call <vilib>:"Clear Errors.vi"("error in (no error)"=w352) -> ("error out"=w351:errorcluster)  [unwired: 5 in, 1 out]
            }
            n120 = call <vilib>:"Clear Errors.vi"("error in (no error)"=w346, "specific error code to clear (0: all)"=w341) -> ("error out"=w348:errorcluster)  [unwired: 4 in, 1 out]
            n121 = call-dynamic "Delacor_lib_QMH_Release Message Queue.vi"("error in"=w348, "Message Queue"=w344) -> ("error out"=w347:errorcluster)  [unwired: 9 in]
            n122 = control-ref of="This VI"() -> (w338:refnum<vi>)
            n123 = call "Handle Exit.vi"("error in"=w333, "Stop Argument"=w339, "Admin in"=w337, "VI reference"=w338) -> ("error out"=w335:errorcluster)  [unwired: 6 in, 1 out]
            n124 = Merge Errors(w347, w335) -> (w345:errorcluster)
            n125 = call "Error Reported.vi"("Error"=w345) -> ()  [unwired: 10 in, 1 out]
          }
          frame Default {
            # "'Default' case only runs if there is a message that isn't defined in any of the other cases.  Output a programming error."
            n126 = call "Module Name--constant.vi"() -> ("Module Name"=w399:string)  [unwired: 11 in]
            n127 = Format Into String(format string="The invalid message string \"%s\" was received in the Message Handling Loop for module \"%s\".", w400, w399) -> (resulting string=w395:string)  [unwired: 2 in, 1 out]
            n128 = call <vilib>:"Error Cluster From Error Code.vi"("show call chain? (False)"=TRUE, "error message (\"\")"=w395, "error code (0)"=1) -> ("error out"=w402:errorcluster)  [unwired: 6 in]
            n129 = Merge Errors(w403, w402) -> (w404:errorcluster)
          }
        }
        n130 = call-dynamic "Delacor_lib_QMH_Error Handler - Message Handling Loop.vi"("error in"=w216, "Message Queue in"=w215) -> ("dup error in"=w217:errorcluster)  [unwired: 8 in, 1 out]
      }
      n131 = while {
        tunnel: w43 -> [w98]
        shift-right: [w101] -> w46
        shift-left: w44 -> [w102]
        tunnel: [w103] -> w48
        tunnel: w42 -> [w99]
        stop <- w100 stop-if-true
        # "Event Handling Loop"
        n132 = event "DQMH_EVENT_MAIN" shown="[13] <Hardware Selection Broadcast Events.Selected RT HW>: User Event" {
          selector: w102 -> [_ _ _ _ _ _ _ _ _ _ _ w166 w175 _ _ w197 w206 _]
          dyn-events: [_ _ _ _ _ _ _ _ _ _ _ w165 w172 _ _ w195 w205 _] -> w101
          timeout: _ -> [_ _ _ _ _ _ _ _ _ _ _ _ _ _ _ _ _ _]
          tunnel: [_ _ _ _ _ _ _ _ _ TRUE ("Discard?") _ _ _ _ _ _ _ _] -> w100
          tunnel: w98 -> [_ _ _ _ w112 _ _ _ _ w131 w145 _ _ _ w187 _ _ w211]
          tunnel: [w110 _ _ _ w113 _ _ w119 _ w141 w147 w167 w178 _ w188 w200 w209 w212] -> w104
          tunnel: w99 -> [_ _ _ _ _ _ _ _ _ _ w144 _ _ _ _ _ _ _]
          event "Simulate EHL Error": Value Change {
            # "#DQMH_HowTo The 'Simulate EHL Error' button  illustrates how the EHL handles errors. This event is instructional in nature and can be removed."
            # "This case simulates an error being generated by the EHL"
            n133 = event-data() -> ()  [unwired: 1 in, 1 out]
            n134 = call "Module Name--constant.vi"() -> ("Module Name"=w107:string)  [unwired: 11 in]
            n135 = Format Into String(format string="Simulated error originating at Event Handling Loop in %s", w107) -> (resulting string=w108:string)  [unwired: 2 in, 1 out]
            n136 = call <vilib>:"Error Cluster From Error Code.vi"("show call chain? (False)"=TRUE, "error message (\"\")"=w108, "error code (0)"=5000) -> ("error out"=w110:errorcluster)  [unwired: 6 in]
          }
          event User Event {
            n137 = event-data() -> ()  [unwired: 1 in, 1 out]
          }
          event User Event {
            n138 = event-data() -> ()  [unwired: 1 in, 6 out]
          }
          event User Event {
            n139 = event-data() -> ()  [unwired: 1 in, 6 out]
          }
          event "Simulate MHL Error": Value Change {
            # "#DQMH_HowTo The 'Simulate MHL Error' button  illustrates how the MHL handles errors. This event is instructional in nature and can be removed."
            # "This case simulates an error being generated by the MHL"
            n140 = event-data() -> ()  [unwired: 1 in, 1 out]
            n141 = call-poly <vilib>:"Delacor_lib_QMH_Enqueue Message (poly).vi"("Message"="Simulate MHL Error", "Message Queue in"=w112) -> ("error out"=w113:errorcluster)  [unwired: 8 in, 1 out]
          }
          event User Event {
            # "Show the panel of this VI, and send a status updated message to let listeners know."
            # "Another Module called the \"Show Panel\" API Method."
            n142 = event-data() -> ()  [unwired: 1 in, 1 out]
            n143 = control-ref of="This VI"() -> (w115:refnum<vi>)
            n144 = call "Open VI Panel.vi"("VI"=w115) -> ()  [unwired: 10 in, 1 out]
            n145 = call "Status Updated.vi"("Status"="Panel shown." ("format string")) -> ()  [unwired: 10 in, 1 out]
          }
          event User Event {
            # "Hide the panel of this VI, and send a status updated message to let listeners know."
            # "Another Module called the \"Hide Panel\" API Method."
            n146 = event-data() -> ()  [unwired: 1 in, 1 out]
            n147 = control-ref of="This VI"() -> (w117:refnum<vi>)
            n148 = call "Hide VI Panel.vi"("VI"=w117) -> ()  [unwired: 10 in, 1 out]
            n149 = call "Status Updated.vi"("Status"="Panel hidden." ("format string")) -> ()  [unwired: 10 in, 1 out]
          }
          event User Event {
            # "Another Module called the \"Get Module Execution Status\" API Method."
            n150 = event-data() -> ()  [unwired: 1 in, 1 out]
            n151 = call "Update Module Execution Status.vi"("Running?"=TRUE) -> ("error out"=w119:errorcluster)  [unwired: 10 in]
          }
          event User Event {
            # "Another Module called the \"Show Diagram\" API Method. This event is used for debugging."
            n152 = event-data() -> ()  [unwired: 1 in, 1 out]
            n153 = disable-structure shown="RUN_TIME_ENGINE==False" {
              frame condition #0 (active) {
                # "functionality not available in exe"
                n154 = invoke on="Invoke Node" class="VI" method="Lock State.Get"() -> (error out=w125:errorcluster, "Get Lock State"=w124:T24, "pwd in cache"=w121:bool)  [unwired: 4 in, 1 out]
                n155 = Equal?(x=T24."Password-protected", y=w124) -> (x = y?=w122:bool)
                n156 = Compound Arithmetic op=AND(w122, invert w121) -> (w120:bool)
                n157 = case shown="False" w120 {
                  tunnel: w125 -> [w128 _]
                  frame False {
                    n158 = property on="Property Node" class="VI"(error in=w128, "BDWin.Open"=TRUE ("Block Diagram Window:Open")) -> ()  [unwired: 1 in, 2 out]
                    n159 = call "Status Updated.vi"("Status"="Block Diagram shown." ("format string")) -> ()  [unwired: 10 in, 1 out]
                  }
                  frame True {
                    # "Password-protected VI, and the password is not in the cache. Do not show the diagram."
                  }
                }
              }
              frame condition #1 {
              }
            }
          }
          event User Event {
            # "The Stop Module Event can get fired from the Exit message in the MHL. The queue gets destroyed in that case. If the queue no longer exists, the Enqueue Exit as a priority message will return error 1. It is safe to ignore, because the module is already exiting."
            # "Another Module called the \"Stop Module\" API Method  or the Message Handling Loop below."
            n160 = event-data() -> ("Origin"=w138:string, "Exit via Stop Module Req?"=w134:bool, "Wait for Module to stop?"=w133:bool)  [unwired: 1 in]
            n161 = local write "Status"(w138) -> ()
            n162 = Bundle By Name(cluster=T25 {"Origin"="", "Exit via Stop Module Req?"=FALSE, "Wait for Module to stop?"=FALSE} ("Stop Argument"), "Exit via Stop Module Req?"=w134, "Wait for Module to stop?"=w133) -> (w132:T25)
            n163 = call-dynamic "Delacor_lib_QMH_Flush Messages.vi"("Message Queue in"=w131) -> ("error out"=w129:errorcluster, "Message Queue out"=w130:refnum<class "Delacor_lib_QMH_Message Queue.lvclass">)  [unwired: 7 in, 2 out]
            n164 = call-poly <vilib>:"Delacor_lib_QMH_Enqueue Message (poly).vi"("Priority Message? (F)"=TRUE, "error in"=w129, "Message Data"=w132, "Message"="Exit", "Message Queue in"=w130) -> ("error out"=w142:errorcluster)  [unwired: 5 in, 1 out]
            n165 = call <vilib>:"Clear Errors.vi"("error in (no error)"=w142, "specific error code to clear (0: all)"=1) -> ("error out"=w141:errorcluster)  [unwired: 4 in, 1 out]
          }
          event Panel Close? {
            w146 = TRUE  # Discard the event, the MHL is responsible for closing and stopping this VI.
            # "Hide the panel or send the 'Exit' message if the user clicks the 'X' on the module main VI panel."
            n166 = event-data() -> ()  [unwired: 1 in, 1 out]
            n167 = property on="Property Node" class="Module Admin"(reference=w144) -> ("Accessors:External Launch"=w143:bool)  [unwired: 1 in, 2 out]
            n168 = case shown="True" w143 {
              tunnel: w145 -> [w149 w158]
              tunnel: [w150 w159] -> w147
              frame True {
                # "If externally launched, clicking the 'X' hides the panel, but doesn't close it."
                n169 = control-ref of="This VI"() -> (w155:refnum<vi>)
                n170 = call "Hide VI Panel.vi"("VI"=w155) -> ("error out"=w153:errorcluster)  [unwired: 10 in]
                n171 = call "Status Updated.vi"("error in"=w153, "Status"="Panel hidden." ("format string")) -> ("error out"=w148:errorcluster)  [unwired: 9 in]
                n172 = call-poly <vilib>:"Delacor_lib_QMH_Enqueue Message (poly).vi"("Priority Message? (F)"=TRUE, "error in"=w148, "Message"="Exit", "Message Queue in"=w149) -> ("error out"=w150:errorcluster)  [unwired: 6 in, 1 out]
              }
              frame False {
                # "If run as a stand-alone VI, clicking the panel 'X' stops the VI."
                n173 = call-poly <vilib>:"Delacor_lib_QMH_Enqueue Message (poly).vi"("Priority Message? (F)"=TRUE, "Message"="Exit", "Message Queue in"=w158) -> ("error out"=w159:errorcluster)  [unwired: 7 in, 1 out]
              }
            }
            n174 = event-data ("Event Filter Node")("Discard?"=w146) -> ()  [unwired: 1 in, 1 out]
          }
          event "Hardware Selection": Value Change {
            n175 = event-data() -> ()  [unwired: 1 in, 5 out]
            n176 = call "Start Module.vi"() -> ("error out"=w164:errorcluster, "Wait for Event Sync?"=w161:bool, "Hardware Selection Broadcast Events"=w163:T9)  [unwired: 8 in, 1 out]
            n177 = register-events "HW-S_REG_EVENTS"(reference=w166, error in=w164, w163) -> (reference out=w165:refnum<event-registration>, error out=w162:errorcluster)  [unwired: 4 in]
            n178 = call "Synchronize Module Events.vi"("error in"=w162, "Wait for Event Sync?"=w161) -> ("error out"=w160:errorcluster)  [unwired: 9 in]
            n179 = case shown="No Error" w160 {
              selector: w160 -> [w168 w170]
              tunnel: [w169 w170] -> w167
              frame No Error {
                n180 = call "Show Panel.vi"("error in"=w168) -> ("error out"=w169:errorcluster)  [unwired: 10 in]
              }
              frame Error {
              }
            }
          }
          event "Automatic Sequence \nConfiguration": Value Change {
            n181 = event-data() -> ()  [unwired: 1 in, 2 out]
            n182 = call "Start Module.vi"() -> ("error out"=w174:errorcluster, "Wait for Event Sync?"=w177:bool, "AS-Configuration Broadcast Events"=w171:T10)  [unwired: 8 in, 1 out]
            n183 = register-events "AS-CON_REG_EVENTS"(reference=w175, error in=w174, w171) -> (reference out=w172:refnum<event-registration>, error out=w173:errorcluster)  [unwired: 4 in]
            n184 = call "Synchronize Module Events.vi"("error in"=w173, "Wait for Event Sync?"=w177) -> ("error out"=w176:errorcluster)  [unwired: 9 in]
            n185 = case shown="No Error" w176 {
              selector: w176 -> [w181 w182]
              tunnel: [w179 w182] -> w178
              frame No Error {
                n186 = call "Hide Panel.vi"("error in"=w181) -> ("error out"=w180:errorcluster)  [unwired: 10 in]
                n187 = call "Show Panel.vi"("error in"=w180) -> ("error out"=w179:errorcluster)  [unwired: 10 in]
              }
              frame Error {
              }
            }
          }
          event User Event {
            w183 = string[] [] ("HW-Name")
            n188 = event-data() -> ()  [unwired: 1 in, 1 out]
            n189 = call "Launch RT Acq.vi"("DO"=T5[] [{"Interface"="DIO", "Interface Data"={"Command"="Configure", "SubCmd"="DO", "Frequency"=500, "Data"=[{"Channel"="Mod1/port0/line0", "Data"=[0], "Identification Name"=""}, {"Channel"="Mod1/port0/line1", "Data"=[0], "Identification Name"=""}, {"Channel"="Mod1/port0/line2", "Data"=[0], "Identification Name"=""}, {"Channel"="Mod1/port0/line3", "Data"=[0], "Identification Name"=""}, {"Channel"="Mod1/port0/line4", "Data"=[0], "Identification Name"=""}, {"Channel"="Mod1/port0/line5", "Data"=[0], "Identification Name"=""}, {"Channel"="Mod1/port0/line6", "Data"=[0], "Identification Name"=""}, {"Channel"="Mod1/port0/line7", "Data"=[0], "Identification Name"=""}, {"Channel"="Mod1/port0/line8", "Data"=[0], "Identification Name"=""}, {"Channel"="Mod1/port0/line9", "Data"=[0], "Identification Name"=""}, {"Channel"="Mod1/port0/line10", "Data"=[0], "Identification Name"=""}, {"Channel"="Mod1/port0/line11", "Data"=[0], "Identification Name"=""}, {"Channel"="Mod1/port0/line12", "Data"=[0], "Identification Name"=""}, {"Channel"="Mod1/port0/line13", "Data"=[0], "Identification Name"=""}, {"Channel"="Mod1/port0/line14", "Data"=[0], "Identification Name"=""}, {"Channel"="Mod1/port0/line15", "Data"=[0], "Identification Name"=""}, {"Channel"="Mod1/port0/line16", "Data"=[0], "Identification Name"=""}, {"Channel"="Mod1/port0/line17", "Data"=[0], "Identification Name"=""}, {"Channel"="Mod1/port0/line18", "Data"=[0], "Identification Name"=""}, {"Channel"="Mod1/port0/line19", "Data"=[0], "Identification Name"=""}, {"Channel"="Mod1/port0/line20", "Data"=[0], "Identification Name"=""}, {"Channel"="Mod1/port0/line21", "Data"=[0], "Identification Name"=""}, {"Channel"="Mod1/port0/line22", "Data"=[0], "Identification Name"=""}, {"Channel"="Mod1/port0/line23", "Data"=[0], "Identification Name"=""}, {"Channel"="Mod1/port0/line24", "Data"=[0], "Identification Name"=""}, {"Channel"="Mod1/port0/line25", "Data"=[0], "Identification Name"=""}, {"Channel"="Mod1/port0/line26", "Data"=[0], "Identification Name"=""}, {"Channel"="Mod1/port0/line27", "Data"=[0], "Identification Name"=""}, {"Channel"="Mod1/port0/line28", "Data"=[0], "Identification Name"=""}, {"Channel"="Mod1/port0/line29", "Data"=[0], "Identification Name"=""}, {"Channel"="Mod1/port0/line30", "Data"=[0], "Identification Name"=""}, {"Channel"="Mod1/port0/line31", "Data"=[0], "Identification Name"=""}]}}, {"Interface"="DIO", "Interface Data"={"Command"="Configure", "SubCmd"="DO", "Frequency"=500, "Data"=[{"Channel"="Mod1/port0/line0", "Data"=[0], "Identification Name"=""}, {"Channel"="Mod1/port0/line1", "Data"=[0], "Identification Name"=""}, {"Channel"="Mod1/port0/line2", "Data"=[0], "Identification Name"=""}, {"Channel"="Mod1/port0/line3", "Data"=[0], "Identification Name"=""}, {"Channel"="Mod1/port0/line4", "Data"=[0], "Identification Name"=""}, {"Channel"="Mod1/port0/line5", "Data"=[0], "Identification Name"=""}, {"Channel"="Mod1/port0/line6", "Data"=[0], "Identification Name"=""}, {"Channel"="Mod1/port0/line7", "Data"=[0], "Identification Name"=""}, {"Channel"="Mod1/port0/line8", "Data"=[0], "Identification Name"=""}, {"Channel"="Mod1/port0/line9", "Data"=[0], "Identification Name"=""}, {"Channel"="Mod1/port0/line10", "Data"=[0], "Identification Name"=""}, {"Channel"="Mod1/port0/line11", "Data"=[0], "Identification Name"=""}, {"Channel"="Mod1/port0/line12", "Data"=[0], "Identification Name"=""}, {"Channel"="Mod1/port0/line13", "Data"=[0], "Identification Name"=""}, {"Channel"="Mod1/port0/line14", "Data"=[0], "Identification Name"=""}, {"Channel"="Mod1/port0/line15", "Data"=[0], "Identification Name"=""}, {"Channel"="Mod1/port0/line16", "Data"=[0], "Identification Name"=""}, {"Channel"="Mod1/port0/line17", "Data"=[0], "Identification Name"=""}, {"Channel"="Mod1/port0/line18", "Data"=[0], "Identification Name"=""}, {"Channel"="Mod1/port0/line19", "Data"=[0], "Identification Name"=""}, {"Channel"="Mod1/port0/line20", "Data"=[0], "Identification Name"=""}, {"Channel"="Mod1/port0/line21", "Data"=[0], "Identification Name"=""}, {"Channel"="Mod1/port0/line22", "Data"=[0], "Identification Name"=""}, {"Channel"="Mod1/port0/line23", "Data"=[0], "Identification Name"=""}, {"Channel"="Mod1/port0/line24", "Data"=[0], "Identification Name"=""}, {"Channel"="Mod1/port0/line25", "Data"=[0], "Identification Name"=""}, {"Channel"="Mod1/port0/line26", "Data"=[0], "Identification Name"=""}, {"Channel"="Mod1/port0/line27", "Data"=[0], "Identification Name"=""}, {"Channel"="Mod1/port0/line28", "Data"=[0], "Identification Name"=""}, {"Channel"="Mod1/port0/line29", "Data"=[0], "Identification Name"=""}, {"Channel"="Mod1/port0/line30", "Data"=[0], "Identification Name"=""}, {"Channel"="Mod1/port0/line31", "Data"=[0], "Identification Name"=""}, {"Channel"="Mod2/port0/line0", "Data"=[0], "Identification Name"=""}, {"Channel"="Mod2/port0/line1", "Data"=[0], "Identification Name"=""}, {"Channel"="Mod2/port0/line2", "Data"=[0], "Identification Name"=""}, {"Channel"="Mod2/port0/line3", "Data"=[0], "Identification Name"=""}, {"Channel"="Mod2/port0/line4", "Data"=[0], "Identification Name"=""}, {"Channel"="Mod2/port0/line5", "Data"=[0], "Identification Name"=""}, {"Channel"="Mod2/port0/line6", "Data"=[0], "Identification Name"=""}, {"Channel"="Mod2/port0/line7", "Data"=[0], "Identification Name"=""}, {"Channel"="Mod2/port0/line8", "Data"=[0], "Identification Name"=""}]}}, {"Interface"="DIO", "Interface Data"={"Command"="Configure", "SubCmd"="DO", "Frequency"=500, "Data"=[{"Channel"="Mod1/port0/line0", "Data"=[0], "Identification Name"=""}, {"Channel"="Mod1/port0/line1", "Data"=[0], "Identification Name"=""}, {"Channel"="Mod1/port0/line2", "Data"=[0], "Identification Name"=""}, {"Channel"="Mod1/port0/line3", "Data"=[0], "Identification Name"=""}, {"Channel"="Mod1/port0/line4", "Data"=[0], "Identification Name"=""}, {"Channel"="Mod1/port0/line5", "Data"=[0], "Identification Name"=""}, {"Channel"="Mod1/port0/line6", "Data"=[], "Identification Name"=""}, {"Channel"="Mod1/port0/line7", "Data"=[0], "Identification Name"=""}, {"Channel"="Mod1/port0/line8", "Data"=[0], "Identification Name"=""}, {"Channel"="Mod1/port0/line9", "Data"=[0], "Identification Name"=""}, {"Channel"="Mod1/port0/line10", "Data"=[0], "Identification Name"=""}, {"Channel"="Mod1/port0/line11", "Data"=[0], "Identification Name"=""}, {"Channel"="Mod1/port0/line12", "Data"=[0], "Identification Name"=""}, {"Channel"="Mod1/port0/line13", "Data"=[0], "Identification Name"=""}, {"Channel"="Mod1/port0/line14", "Data"=[0], "Identification Name"=""}, {"Channel"="Mod1/port0/line15", "Data"=[0], "Identification Name"=""}, {"Channel"="Mod1/port0/line16", "Data"=[0], "Identification Name"=""}, {"Channel"="Mod1/port0/line17", "Data"=[0], "Identification Name"=""}, {"Channel"="Mod1/port0/line18", "Data"=[0], "Identification Name"=""}, {"Channel"="Mod1/port0/line19", "Data"=[0], "Identification Name"=""}, {"Channel"="Mod1/port0/line20", "Data"=[0], "Identification Name"=""}, {"Channel"="Mod1/port0/line21", "Data"=[0], "Identification Name"=""}, {"Channel"="Mod1/port0/line22", "Data"=[0], "Identification Name"=""}, {"Channel"="Mod1/port0/line23", "Data"=[0], "Identification Name"=""}, {"Channel"="Mod1/port0/line24", "Data"=[0], "Identification Name"=""}, {"Channel"="Mod1/port0/line25", "Data"=[0], "Identification Name"=""}, {"Channel"="Mod1/port0/line26", "Data"=[0], "Identification Name"=""}, {"Channel"="Mod1/port0/line27", "Data"=[0], "Identification Name"=""}, {"Channel"="Mod1/port0/line28", "Data"=[0], "Identification Name"=""}, {"Channel"="Mod1/port0/line29", "Data"=[0], "Identification Name"=""}, {"Channel"="Mod1/port0/line30", "Data"=[0], "Identification Name"=""}, {"Channel"="Mod1/port0/line31", "Data"=[0], "Identification Name"=""}]}}, {"Interface"="DIO", "Interface Data"={"Command"="Configure", "SubCmd"="DO", "Frequency"=500, "Data"=[{"Channel"="Mod1/port0/line0", "Data"=[0], "Identification Name"=""}, {"Channel"="Mod1/port0/line1", "Data"=[0], "Identification Name"=""}, {"Channel"="Mod1/port0/line2", "Data"=[0], "Identification Name"=""}, {"Channel"="Mod1/port0/line3", "Data"=[0], "Identification Name"=""}, {"Channel"="Mod1/port0/line4", "Data"=[0], "Identification Name"=""}, {"Channel"="Mod1/port0/line5", "Data"=[0], "Identification Name"=""}, {"Channel"="Mod1/port0/line6", "Data"=[0], "Identification Name"=""}, {"Channel"="Mod1/port0/line7", "Data"=[0], "Identification Name"=""}, {"Channel"="Mod1/port0/line8", "Data"=[0], "Identification Name"=""}, {"Channel"="Mod1/port0/line9", "Data"=[0], "Identification Name"=""}, {"Channel"="Mod1/port0/line10", "Data"=[0], "Identification Name"=""}, {"Channel"="Mod1/port0/line11", "Data"=[0], "Identification Name"=""}, {"Channel"="Mod1/port0/line12", "Data"=[0], "Identification Name"=""}, {"Channel"="Mod1/port0/line13", "Data"=[0], "Identification Name"=""}, {"Channel"="Mod1/port0/line14", "Data"=[0], "Identification Name"=""}, {"Channel"="Mod1/port0/line15", "Data"=[0], "Identification Name"=""}, {"Channel"="Mod1/port0/line16", "Data"=[0], "Identification Name"=""}, {"Channel"="Mod1/port0/line17", "Data"=[0], "Identification Name"=""}, {"Channel"="Mod1/port0/line18", "Data"=[0], "Identification Name"=""}, {"Channel"="Mod1/port0/line19", "Data"=[0], "Identification Name"=""}, {"Channel"="Mod1/port0/line20", "Data"=[0], "Identification Name"=""}, {"Channel"="Mod1/port0/line21", "Data"=[0], "Identification Name"=""}, {"Channel"="Mod1/port0/line22", "Data"=[0], "Identification Name"=""}, {"Channel"="Mod1/port0/line23", "Data"=[0], "Identification Name"=""}, {"Channel"="Mod1/port0/line24", "Data"=[0], "Identification Name"=""}, {"Channel"="Mod1/port0/line25", "Data"=[0], "Identification Name"=""}, {"Channel"="Mod1/port0/line26", "Data"=[0], "Identification Name"=""}, {"Channel"="Mod1/port0/line27", "Data"=[0], "Identification Name"=""}, {"Channel"="Mod1/port0/line28", "Data"=[0], "Identification Name"=""}, {"Channel"="Mod1/port0/line29", "Data"=[0], "Identification Name"=""}, {"Channel"="Mod1/port0/line30", "Data"=[0], "Identification Name"=""}, {"Channel"="Mod1/port0/line31", "Data"=[0], "Identification Name"=""}]}}, {"Interface"="DIO", "Interface Data"={"Command"="Configure", "SubCmd"="DO", "Frequency"=500, "Data"=[{"Channel"="Mod1/port0/line0", "Data"=[0], "Identification Name"=""}, {"Channel"="Mod1/port0/line1", "Data"=[0], "Identification Name"=""}, {"Channel"="Mod1/port0/line2", "Data"=[0], "Identification Name"=""}, {"Channel"="Mod1/port0/line3", "Data"=[0], "Identification Name"=""}, {"Channel"="Mod1/port0/line4", "Data"=[0], "Identification Name"=""}, {"Channel"="Mod1/port0/line5", "Data"=[0], "Identification Name"=""}, {"Channel"="Mod1/port0/line6", "Data"=[0], "Identification Name"=""}, {"Channel"="Mod1/port0/line7", "Data"=[0], "Identification Name"=""}, {"Channel"="Mod1/port0/line8", "Data"=[0], "Identification Name"=""}, {"Channel"="Mod1/port0/line9", "Data"=[0], "Identification Name"=""}, {"Channel"="Mod1/port0/line10", "Data"=[0], "Identification Name"=""}, {"Channel"="Mod1/port0/line11", "Data"=[0], "Identification Name"=""}, {"Channel"="Mod1/port0/line12", "Data"=[0], "Identification Name"=""}, {"Channel"="Mod1/port0/line13", "Data"=[0], "Identification Name"=""}, {"Channel"="Mod1/port0/line14", "Data"=[0], "Identification Name"=""}, {"Channel"="Mod1/port0/line15", "Data"=[0], "Identification Name"=""}, {"Channel"="Mod1/port0/line16", "Data"=[0], "Identification Name"=""}, {"Channel"="Mod1/port0/line17", "Data"=[0], "Identification Name"=""}, {"Channel"="Mod1/port0/line18", "Data"=[0], "Identification Name"=""}, {"Channel"="Mod1/port0/line19", "Data"=[0], "Identification Name"=""}, {"Channel"="Mod1/port0/line20", "Data"=[0], "Identification Name"=""}, {"Channel"="Mod1/port0/line21", "Data"=[0], "Identification Name"=""}, {"Channel"="Mod1/port0/line22", "Data"=[0], "Identification Name"=""}, {"Channel"="Mod1/port0/line23", "Data"=[0], "Identification Name"=""}, {"Channel"="Mod1/port0/line24", "Data"=[0], "Identification Name"=""}, {"Channel"="Mod1/port0/line25", "Data"=[0], "Identification Name"=""}, {"Channel"="Mod1/port0/line26", "Data"=[0], "Identification Name"=""}, {"Channel"="Mod1/port0/line27", "Data"=[0], "Identification Name"=""}, {"Channel"="Mod1/port0/line28", "Data"=[0], "Identification Name"=""}, {"Channel"="Mod1/port0/line29", "Data"=[0], "Identification Name"=""}, {"Channel"="Mod1/port0/line30", "Data"=[0], "Identification Name"=""}, {"Channel"="Mod1/port0/line31", "Data"=[0], "Identification Name"=""}]}}, {"Interface"="DIO", "Interface Data"={"Command"="Configure", "SubCmd"="DO", "Frequency"=500, "Data"=[{"Channel"="Mod1/port0/line0", "Data"=[0], "Identification Name"=""}, {"Channel"="Mod1/port0/line1", "Data"=[0], "Identification Name"=""}, {"Channel"="Mod1/port0/line2", "Data"=[0], "Identification Name"=""}, {"Channel"="Mod1/port0/line3", "Data"=[0], "Identification Name"=""}, {"Channel"="Mod1/port0/line4", "Data"=[0], "Identification Name"=""}, {"Channel"="Mod1/port0/line5", "Data"=[0], "Identification Name"=""}, {"Channel"="Mod1/port0/line6", "Data"=[0], "Identification Name"=""}, {"Channel"="Mod1/port0/line7", "Data"=[0], "Identification Name"=""}, {"Channel"="Mod1/port0/line8", "Data"=[0], "Identification Name"=""}, {"Channel"="Mod1/port0/line9", "Data"=[0], "Identification Name"=""}, {"Channel"="Mod1/port0/line10", "Data"=[0], "Identification Name"=""}, {"Channel"="Mod1/port0/line11", "Data"=[0], "Identification Name"=""}, {"Channel"="Mod1/port0/line12", "Data"=[0], "Identification Name"=""}, {"Channel"="Mod1/port0/line13", "Data"=[0], "Identification Name"=""}, {"Channel"="Mod1/port0/line14", "Data"=[0], "Identification Name"=""}, {"Channel"="Mod1/port0/line15", "Data"=[0], "Identification Name"=""}, {"Channel"="Mod1/port0/line16", "Data"=[0], "Identification Name"=""}, {"Channel"="Mod1/port0/line17", "Data"=[0], "Identification Name"=""}, {"Channel"="Mod1/port0/line18", "Data"=[0], "Identification Name"=""}, {"Channel"="Mod1/port0/line19", "Data"=[0], "Identification Name"=""}, {"Channel"="Mod1/port0/line20", "Data"=[0], "Identification Name"=""}, {"Channel"="Mod1/port0/line21", "Data"=[0], "Identification Name"=""}, {"Channel"="Mod1/port0/line22", "Data"=[0], "Identification Name"=""}, {"Channel"="Mod1/port0/line23", "Data"=[0], "Identification Name"=""}, {"Channel"="Mod1/port0/line24", "Data"=[0], "Identification Name"=""}, {"Channel"="Mod1/port0/line25", "Data"=[0], "Identification Name"=""}, {"Channel"="Mod1/port0/line26", "Data"=[0], "Identification Name"=""}, {"Channel"="Mod1/port0/line27", "Data"=[0], "Identification Name"=""}, {"Channel"="Mod1/port0/line28", "Data"=[0], "Identification Name"=""}, {"Channel"="Mod1/port0/line29", "Data"=[0], "Identification Name"=""}, {"Channel"="Mod1/port0/line30", "Data"=[0], "Identification Name"=""}, {"Channel"="Mod1/port0/line31", "Data"=[0], "Identification Name"=""}, {"Channel"="Mod2/port0/line0", "Data"=[0], "Identification Name"=""}, {"Channel"="Mod2/port0/line1", "Data"=[0], "Identification Name"=""}, {"Channel"="Mod2/port0/line2", "Data"=[0], "Identification Name"=""}, {"Channel"="Mod2/port0/line3", "Data"=[0], "Identification Name"=""}, {"Channel"="Mod2/port0/line4", "Data"=[0], "Identification Name"=""}, {"Channel"="Mod2/port0/line5", "Data"=[0], "Identification Name"=""}, {"Channel"="Mod2/port0/line6", "Data"=[0], "Identification Name"=""}, {"Channel"="Mod2/port0/line7", "Data"=[0], "Identification Name"=""}, {"Channel"="Mod2/port0/line8", "Data"=[0], "Identification Name"=""}, {"Channel"="Mod2/port0/line9", "Data"=[0], "Identification Name"=""}, {"Channel"="Mod2/port0/line10", "Data"=[0], "Identification Name"=""}, {"Channel"="Mod2/port0/line11", "Data"=[0], "Identification Name"=""}, {"Channel"="Mod2/port0/line12", "Data"=[0], "Identification Name"=""}, {"Channel"="Mod2/port0/line13", "Data"=[0], "Identification Name"=""}, {"Channel"="Mod2/port0/line14", "Data"=[0], "Identification Name"=""}, {"Channel"="Mod2/port0/line15", "Data"=[0], "Identification Name"=""}, {"Channel"="Mod2/port0/line16", "Data"=[0], "Identification Name"=""}, {"Channel"="Mod2/port0/line17", "Data"=[0], "Identification Name"=""}, {"Channel"="Mod2/port0/line18", "Data"=[0], "Identification Name"=""}, {"Channel"="Mod2/port0/line19", "Data"=[0], "Identification Name"=""}, {"Channel"="Mod2/port0/line20", "Data"=[0], "Identification Name"=""}, {"Channel"="Mod2/port0/line21", "Data"=[0], "Identification Name"=""}, {"Channel"="Mod2/port0/line22", "Data"=[0], "Identification Name"=""}, {"Channel"="Mod2/port0/line23", "Data"=[0], "Identification Name"=""}, {"Channel"="Mod2/port0/line24", "Data"=[0], "Identification Name"=""}, {"Channel"="Mod2/port0/line25", "Data"=[0], "Identification Name"=""}, {"Channel"="Mod2/port0/line26", "Data"=[0], "Identification Name"=""}, {"Channel"="Mod2/port0/line27", "Data"=[0], "Identification Name"=""}, {"Channel"="Mod2/port0/line28", "Data"=[0], "Identification Name"=""}, {"Channel"="Mod2/port0/line29", "Data"=[0], "Identification Name"=""}, {"Channel"="Mod2/port0/line30", "Data"=[0], "Identification Name"=""}, {"Channel"="Mod2/port0/line31", "Data"=[0], "Identification Name"=""}]}}], "DI"=T5[] [{"Interface"="DIO", "Interface Data"={"Command"="Configure", "SubCmd"="DI", "Frequency"=500, "Data"=[{"Channel"="Mod3/port0/line0", "Data"=[0], "Identification Name"=""}, {"Channel"="Mod3/port0/line1", "Data"=[0], "Identification Name"=""}, {"Channel"="Mod3/port0/line2", "Data"=[0], "Identification Name"=""}, {"Channel"="Mod3/port0/line3", "Data"=[0], "Identification Name"=""}, {"Channel"="Mod3/port0/line4", "Data"=[0], "Identification Name"=""}, {"Channel"="Mod3/port0/line5", "Data"=[0], "Identification Name"=""}, {"Channel"="Mod3/port0/line6", "Data"=[0], "Identification Name"=""}, {"Channel"="Mod3/port0/line7", "Data"=[0], "Identification Name"=""}, {"Channel"="Mod3/port0/line8", "Data"=[0], "Identification Name"=""}, {"Channel"="Mod3/port0/line9", "Data"=[0], "Identification Name"=""}, {"Channel"="Mod3/port0/line10", "Data"=[0], "Identification Name"=""}, {"Channel"="Mod3/port0/line11", "Data"=[0], "Identification Name"=""}, {"Channel"="Mod3/port0/line12", "Data"=[0], "Identification Name"=""}, {"Channel"="Mod3/port0/line13", "Data"=[0], "Identification Name"=""}, {"Channel"="Mod3/port0/line14", "Data"=[0], "Identification Name"=""}, {"Channel"="Mod3/port0/line15", "Data"=[0], "Identification Name"=""}, {"Channel"="Mod3/port0/line16", "Data"=[0], "Identification Name"=""}, {"Channel"="Mod3/port0/line17", "Data"=[0], "Identification Name"=""}, {"Channel"="Mod3/port0/line18", "Data"=[0], "Identification Name"=""}, {"Channel"="Mod3/port0/line19", "Data"=[0], "Identification Name"=""}, {"Channel"="Mod3/port0/line20", "Data"=[0], "Identification Name"=""}, {"Channel"="Mod3/port0/line21", "Data"=[0], "Identification Name"=""}, {"Channel"="Mod3/port0/line22", "Data"=[0], "Identification Name"=""}, {"Channel"="Mod3/port0/line23", "Data"=[0], "Identification Name"=""}, {"Channel"="Mod3/port0/line24", "Data"=[0], "Identification Name"=""}, {"Channel"="Mod3/port0/line25", "Data"=[0], "Identification Name"=""}, {"Channel"="Mod3/port0/line26", "Data"=[0], "Identification Name"=""}, {"Channel"="Mod3/port0/line27", "Data"=[0], "Identification Name"=""}, {"Channel"="Mod3/port0/line28", "Data"=[0], "Identification Name"=""}, {"Channel"="Mod3/port0/line29", "Data"=[0], "Identification Name"=""}, {"Channel"="Mod3/port0/line30", "Data"=[0], "Identification Name"=""}, {"Channel"="Mod3/port0/line31", "Data"=[0], "Identification Name"=""}, {"Channel"="Mod4/port0/line0", "Data"=[0], "Identification Name"=""}, {"Channel"="Mod4/port0/line1", "Data"=[0], "Identification Name"=""}, {"Channel"="Mod4/port0/line2", "Data"=[0], "Identification Name"=""}, {"Channel"="Mod4/port0/line3", "Data"=[0], "Identification Name"=""}, {"Channel"="Mod4/port0/line4", "Data"=[0], "Identification Name"=""}, {"Channel"="Mod4/port0/line5", "Data"=[0], "Identification Name"=""}, {"Channel"="Mod4/port0/line6", "Data"=[0], "Identification Name"=""}, {"Channel"="Mod4/port0/line7", "Data"=[0], "Identification Name"=""}, {"Channel"="Mod4/port0/line8", "Data"=[0], "Identification Name"=""}, {"Channel"="Mod4/port0/line9", "Data"=[0], "Identification Name"=""}, {"Channel"="Mod4/port0/line10", "Data"=[0], "Identification Name"=""}, {"Channel"="Mod4/port0/line11", "Data"=[0], "Identification Name"=""}, {"Channel"="Mod4/port0/line12", "Data"=[0], "Identification Name"=""}, {"Channel"="Mod4/port0/line13", "Data"=[0], "Identification Name"=""}, {"Channel"="Mod4/port0/line14", "Data"=[0], "Identification Name"=""}, {"Channel"="Mod4/port0/line15", "Data"=[0], "Identification Name"=""}, {"Channel"="Mod4/port0/line16", "Data"=[0], "Identification Name"=""}, {"Channel"="Mod4/port0/line17", "Data"=[0], "Identification Name"=""}, {"Channel"="Mod4/port0/line18", "Data"=[0], "Identification Name"=""}, {"Channel"="Mod4/port0/line19", "Data"=[0], "Identification Name"=""}, {"Channel"="Mod4/port0/line20", "Data"=[0], "Identification Name"=""}, {"Channel"="Mod4/port0/line21", "Data"=[0], "Identification Name"=""}, {"Channel"="Mod4/port0/line22", "Data"=[0], "Identification Name"=""}, {"Channel"="Mod4/port0/line23", "Data"=[0], "Identification Name"=""}, {"Channel"="Mod4/port0/line24", "Data"=[0], "Identification Name"=""}, {"Channel"="Mod4/port0/line25", "Data"=[0], "Identification Name"=""}, {"Channel"="Mod4/port0/line26", "Data"=[0], "Identification Name"=""}, {"Channel"="Mod4/port0/line27", "Data"=[0], "Identification Name"=""}, {"Channel"="Mod4/port0/line28", "Data"=[0], "Identification Name"=""}, {"Channel"="Mod4/port0/line29", "Data"=[0], "Identification Name"=""}, {"Channel"="Mod4/port0/line30", "Data"=[0], "Identification Name"=""}, {"Channel"="Mod4/port0/line31", "Data"=[0], "Identification Name"=""}]}}, {"Interface"="DIO", "Interface Data"={"Command"="", "SubCmd"="DI", "Frequency"=500, "Data"=[]}}, {"Interface"="DIO", "Interface Data"={"Command"="Configure", "SubCmd"="DI", "Frequency"=500, "Data"=[{"Channel"="Mod3/port0/line0", "Data"=[0], "Identification Name"=""}, {"Channel"="Mod3/port0/line1", "Data"=[0], "Identification Name"=""}, {"Channel"="Mod3/port0/line2", "Data"=[0], "Identification Name"=""}, {"Channel"="Mod3/port0/line3", "Data"=[0], "Identification Name"=""}, {"Channel"="Mod3/port0/line4", "Data"=[0], "Identification Name"=""}, {"Channel"="Mod3/port0/line5", "Data"=[0], "Identification Name"=""}, {"Channel"="Mod3/port0/line6", "Data"=[0], "Identification Name"=""}, {"Channel"="Mod3/port0/line7", "Data"=[0], "Identification Name"=""}, {"Channel"="Mod3/port0/line8", "Data"=[0], "Identification Name"=""}, {"Channel"="Mod3/port0/line9", "Data"=[0], "Identification Name"=""}, {"Channel"="Mod3/port0/line10", "Data"=[0], "Identification Name"=""}, {"Channel"="Mod3/port0/line11", "Data"=[0], "Identification Name"=""}, {"Channel"="Mod3/port0/line12", "Data"=[0], "Identification Name"=""}, {"Channel"="Mod3/port0/line13", "Data"=[0], "Identification Name"=""}, {"Channel"="Mod3/port0/line14", "Data"=[0], "Identification Name"=""}, {"Channel"="Mod3/port0/line15", "Data"=[0], "Identification Name"=""}, {"Channel"="Mod3/port0/line16", "Data"=[0], "Identification Name"=""}, {"Channel"="Mod3/port0/line17", "Data"=[0], "Identification Name"=""}, {"Channel"="Mod3/port0/line18", "Data"=[0], "Identification Name"=""}, {"Channel"="Mod3/port0/line19", "Data"=[0], "Identification Name"=""}, {"Channel"="Mod3/port0/line20", "Data"=[0], "Identification Name"=""}, {"Channel"="Mod3/port0/line21", "Data"=[0], "Identification Name"=""}, {"Channel"="Mod3/port0/line22", "Data"=[0], "Identification Name"=""}, {"Channel"="Mod3/port0/line23", "Data"=[0], "Identification Name"=""}, {"Channel"="Mod3/port0/line24", "Data"=[0], "Identification Name"=""}, {"Channel"="Mod3/port0/line25", "Data"=[0], "Identification Name"=""}, {"Channel"="Mod3/port0/line26", "Data"=[0], "Identification Name"=""}, {"Channel"="Mod3/port0/line27", "Data"=[0], "Identification Name"=""}, {"Channel"="Mod3/port0/line28", "Data"=[0], "Identification Name"=""}, {"Channel"="Mod3/port0/line29", "Data"=[0], "Identification Name"=""}, {"Channel"="Mod3/port0/line30", "Data"=[0], "Identification Name"=""}, {"Channel"="Mod3/port0/line31", "Data"=[0], "Identification Name"=""}, {"Channel"="Mod4/port0/line0", "Data"=[0], "Identification Name"=""}, {"Channel"="Mod4/port0/line1", "Data"=[0], "Identification Name"=""}, {"Channel"="Mod4/port0/line2", "Data"=[0], "Identification Name"=""}, {"Channel"="Mod4/port0/line3", "Data"=[0], "Identification Name"=""}, {"Channel"="Mod4/port0/line4", "Data"=[0], "Identification Name"=""}, {"Channel"="Mod4/port0/line5", "Data"=[0], "Identification Name"=""}, {"Channel"="Mod4/port0/line6", "Data"=[0], "Identification Name"=""}, {"Channel"="Mod4/port0/line7", "Data"=[0], "Identification Name"=""}, {"Channel"="Mod4/port0/line8", "Data"=[0], "Identification Name"=""}, {"Channel"="Mod4/port0/line9", "Data"=[0], "Identification Name"=""}, {"Channel"="Mod4/port0/line10", "Data"=[0], "Identification Name"=""}, {"Channel"="Mod4/port0/line11", "Data"=[0], "Identification Name"=""}, {"Channel"="Mod4/port0/line12", "Data"=[0], "Identification Name"=""}, {"Channel"="Mod4/port0/line13", "Data"=[0], "Identification Name"=""}, {"Channel"="Mod4/port0/line14", "Data"=[0], "Identification Name"=""}, {"Channel"="Mod4/port0/line15", "Data"=[0], "Identification Name"=""}, {"Channel"="Mod4/port0/line16", "Data"=[0], "Identification Name"=""}, {"Channel"="Mod4/port0/line17", "Data"=[0], "Identification Name"=""}, {"Channel"="Mod4/port0/line18", "Data"=[0], "Identification Name"=""}, {"Channel"="Mod4/port0/line19", "Data"=[0], "Identification Name"=""}, {"Channel"="Mod4/port0/line20", "Data"=[0], "Identification Name"=""}, {"Channel"="Mod4/port0/line21", "Data"=[0], "Identification Name"=""}, {"Channel"="Mod4/port0/line22", "Data"=[0], "Identification Name"=""}, {"Channel"="Mod4/port0/line23", "Data"=[0], "Identification Name"=""}, {"Channel"="Mod4/port0/line24", "Data"=[0], "Identification Name"=""}, {"Channel"="Mod4/port0/line25", "Data"=[0], "Identification Name"=""}, {"Channel"="Mod4/port0/line26", "Data"=[0], "Identification Name"=""}, {"Channel"="Mod4/port0/line27", "Data"=[0], "Identification Name"=""}, {"Channel"="Mod4/port0/line28", "Data"=[0], "Identification Name"=""}, {"Channel"="Mod4/port0/line29", "Data"=[0], "Identification Name"=""}, {"Channel"="Mod4/port0/line30", "Data"=[0], "Identification Name"=""}, {"Channel"="Mod4/port0/line31", "Data"=[0], "Identification Name"=""}]}}, {"Interface"="DIO", "Interface Data"={"Command"="Configure", "SubCmd"="DI", "Frequency"=500, "Data"=[]}}, {"Interface"="DIO", "Interface Data"={"Command"="Configure", "SubCmd"="DI", "Frequency"=500, "Data"=[]}}, {"Interface"="DIO", "Interface Data"={"Command"="Configure", "SubCmd"="DI", "Frequency"=500, "Data"=[]}}], "AI"="AI 2", "HW-IP"=w183, "HW-Name"=w183) -> ()  [unwired: 6 in, 1 out]
          }
          event Menu Selection (User) {
            n190 = event-data() -> ("ItemTag"=w189:string)  [unwired: 1 in]
            n191 = case shown="\"Stop c-RIO Application\", Default" w189 {
              tunnel: [w191 _] -> w188
              tunnel: w187 -> [w190 _]
              frame "Stop c-RIO Application", Default {
                n192 = call-poly <vilib>:"Delacor_lib_QMH_Enqueue Message (poly).vi"("Message"="Stop RT Application's", "Message Queue in"=w190) -> ("error out"=w191:errorcluster)  [unwired: 8 in, 1 out]
              }
              frame "Stop sb-RIO Application" {
              }
            }
          }
          event "Test  configuration": Value Change {
            n193 = event-data() -> ()  [unwired: 1 in, 1 out]
            n194 = call "Start Module.vi"() -> ("error out"=w196:errorcluster, "Wait for Event Sync?"=w199:bool, "Test Configuration Broadcast Events"=w194:T8)  [unwired: 8 in, 1 out]
            n195 = register-events "Test Config-Reg"(reference=w197, error in=w196, w194) -> (reference out=w195:refnum<event-registration>, error out=w198:errorcluster)  [unwired: 4 in]
            n196 = call "Synchronize Module Events.vi"("error in"=w198, "Wait for Event Sync?"=w199) -> ("error out"=w193:errorcluster)  [unwired: 9 in]
            n197 = call "Hide Panel.vi"("error in"=w193) -> ("error out"=w201:errorcluster)  [unwired: 10 in]
            n198 = call "Show Panel.vi"("error in"=w201) -> ("error out"=w200:errorcluster)  [unwired: 10 in]
          }
          event "Acquisition Module Configuration": Value Change {
            n199 = event-data() -> ()  [unwired: 1 in, 1 out]
            n200 = call "Start Module.vi"() -> ("error out"=w204:errorcluster, "Wait for Event Sync?"=w208:bool, "Configuration Broadcast Events"=w202:T11)  [unwired: 8 in, 1 out]
            n201 = register-events "Configuration-Reg"(reference=w206, error in=w204, w202) -> (reference out=w205:refnum<event-registration>, error out=w207:errorcluster)  [unwired: 4 in]
            n202 = call "Synchronize Module Events.vi"("error in"=w207, "Wait for Event Sync?"=w208) -> ("error out"=w203:errorcluster)  [unwired: 9 in]
            n203 = call "Hide Panel.vi"("error in"=w203) -> ("error out"=w210:errorcluster)  [unwired: 10 in]
            n204 = call "Show Panel.vi"("error in"=w210) -> ("error out"=w209:errorcluster)  [unwired: 10 in]
          }
          event "Offline Analysis": Value Change {
            n205 = event-data() -> ()  [unwired: 1 in, 1 out]
            n206 = call-poly <vilib>:"Delacor_lib_QMH_Enqueue Message (poly).vi"("Message"="Launch Offline Analysis", "Message Queue in"=w211) -> ("error out"=w212:errorcluster)  [unwired: 8 in, 1 out]
          }
        }
        n207 = call-dynamic "Delacor_lib_QMH_Error Handler - Event Handling Loop.vi"("error in"=w104, "Message Queue in"=w98) -> ("dup error in"=w103:errorcluster)  [unwired: 8 in, 1 out]
      }
      n208 = call <vilib>:"Stop Helper Loop.vi"("Helper Loop Periodic Timing in"=w36) -> ()  [unwired: 1 out]
      n209 = Unregister For Events(event registration refnum=w40) -> ()  [unwired: 1 in, 1 out]
    }
    frame Error {
      # "Synchronize Caller Events.vi will inform Start Module.vi that the module has launched and will let the code calling Start Module.vi register for broadcasts and would permit the caller receive the broadcast that an error occurred at launch time."
      n210 = call-dynamic "Delacor_lib_QMH_Release Message Queue.vi"("error in"=w412, "Message Queue"=w405) -> ("error out"=w411:errorcluster)  [unwired: 9 in]
      n211 = call "Synchronize Caller Events.vi"("Singleton Module Admin in"=w406) -> ("error out"=w413:errorcluster)  [unwired: 9 in, 1 out]
      n212 = call "Module Name--constant.vi"() -> ("Module Name"=w409:string)  [unwired: 11 in]
      n213 = Format Into String(format string="An error occurred during initialization. %s is no longer running.", w409) -> (resulting string=w407:string)  [unwired: 2 in, 1 out]
      n214 = Merge Errors(w411, w413) -> (w414:errorcluster)
      n215 = call "Error Reported.vi"("Additional Information"=w407, "Error"=w414) -> ()  [unwired: 9 in, 1 out]
    }
  }
  n216 = Merge Errors(w26, w29) -> (w25:errorcluster)
  n217 = call "Close Module.vi"("error in"=w25, "Module Admin in"=w21) -> ("error out"=w27:errorcluster, "External Launch"=w15:bool, "Module Admin out"=w16:refnum<class "Delacor_lib_QMH_Module Admin.lvclass">)  [unwired: 7 in]
  n218 = disable-structure shown="Disabled" {
    frame Disabled {
      n219 = call "RT Module ID.vi"() -> ()  [unwired: 12 in, 4 out]
    }
    frame Enabled {
    }
  }
  n220 = Unregister For Events(event registration refnum=w20, error in=w27) -> (error out=w24:errorcluster)
  n221 = case "External Launch?" shown="False" w15 {
    tunnel: w24 -> [w415 w417]
    tunnel: [w415 w416] -> w11
    frame False {
    }
    frame True {
      n222 = case shown="No Error" w417 {
        selector: w417 -> [w418 w419]
        tunnel: [w418 w419] -> w416
        frame No Error {
          n223 = invoke on="Invoke Node" class="VI" method="FP.Close"() -> ()  [unwired: 3 in, 3 out]
        }
        frame Error {
          n224 = invoke on="Invoke Node" class="VI" method="FP.Open"("Activate"=TRUE ("Activate?")) -> ()  [unwired: 4 in, 5 out]
        }
      }
    }
  }
  n225 = local write "Module Admin"(w16) -> ()
  n226 = disable-structure shown="RUN_TIME_ENGINE==True" {
    disable-tunnel: w11 -> [w421 w423]
    disable-tunnel: [w421 w423] -> w10
    frame condition #0 (active) {
    }
    frame condition #1 {
      n227 = Quit LabVIEW(quit? (T)=TRUE) -> ()
    }
  }
  "error out" <- w10
